vi "Lockin-4461 -Patrick -State 2.0.vi"(10 "IV Curve Mode":bool, 11 "Channels: AO":T8={"AO amp (V)"=[0.0, 0.0, 0.0, 0.0, 0.0, 0.0, 0.0, 0.0], "AO DC (V)"=[0.0, 0.0, 0.0, 0.0, 0.0, 0.0, 0.0, 0.0], "AO f (Hz)"=[13.0, 13.0, 13.0, 13.0, 13.0, 13.0, 13.0, 13.0], "AO phi (deg)"=[0.0, 0.0, 0.0, 0.0, 0.0, 0.0, 0.0, 0.0], "function"=[enum."Sine Wave", enum."Sine Wave", enum."Sine Wave", enum."Sine Wave", enum."Sine Wave", enum."Sine Wave", enum."Sine Wave", enum."Sine Wave"]} {"AO f (Hz)" min=0.001 max=10000.0; "AO DC (V)" format="%#_6p"; "AO amp (V)" format="%#_6p"}) -> ()   [LabVIEW 2013]
uses:
  <vilib>/Analysis/4window.llb/windowTd.ctl
  <vilib>/measure/maspectr.llb/Power Spectrum and PSD Export Mode.ctl
  <vilib>/Utility/error.llb/DialogType.ctl
  <vilib>/Analysis/baseanly.llb/Mean (DBL).vi
  <vilib>/Analysis/2dsp.llb/Decimate (single shot).vi
  <vilib>/Analysis/2dsp.llb/Decimate (single shot, DBL).vi
  <userlib>/_OpenG.lib/array/array.llb/Empty 1D Array (Variant)__ogtk.vi
  <vilib>/Platform/browser.llb/Open URL in Default Browser (string).vi
  <userlib>/_OpenG.lib/error/error.llb/Filter Error Codes (Array)__ogtk.vi
  <userlib>/_OpenG.lib/array/array.llb/Empty 1D Array (DBL)__ogtk.vi
  <vilib>/measure/maspectr.llb/FFT Power Spectrum and PSD for N Chan.vi
  <vilib>/Waveform/WDTOps.llb/WDT Waveform to XY Pairs DBL.vi
  <vilib>/measure/NI_MAPro.lvlib
  <vilib>/Analysis/NI_AALBase.lvlib
  <vilib>/Utility/config.llb/NI_LVConfig.lvlib
  <vilib>/Analysis/NI_AALPro.lvlib
panel:
  in  "Tab Control 3":enum32{"Page 1"}(tab)
  in  "Notes":string
  in  "Path":path=path "C:/Data/lockin"
  in  "EXIT":bool
  in  "RESET":bool
  in  "Save Data":bool
  out "X or R":dbl=0.0008668764236983905 caption="X or R: Current (A) or Voltage (V)" format="%#.3p"
  out "Y or Theta":dbl=-50.403184981183465 caption="Y or Theta: Current (A) or Voltage (V)" format="%.3p"
  in  "Display":enum16{"X and Y", "R and Theta"}(ring)=enum."R and Theta"
  in  "Channel":dbl min=0.0 max=7.0 step=1.0
  in  "Remote Mode":bool
  out "time and date":string="22:19:38.7   2016-11-29"
  out "DAQ mode string":string="None"
  out "time since trigger":dbl
  in  "mean":dbl[](array[numeric])=[0.003634816212724108, -0.004266485588942877, 0.0008988807363483967, 0.001923221656187443, -0.0014081863319705614, 0.0031806607498407746, -0.004900231349882742, 0.00649024630273491]
  in  "Tab Control 2":T1(tab)
  in  "Output signals?":bool
  out "Signals Graph":waveform(dbl)[](graph)=[{"t0"=timestamp(3563320778.6520257 s since 1904-01-01), "dt"=1.0, "Y"=array[10000 elements]}, {"t0"=timestamp(3563320778.6520257 s since 1904-01-01), "dt"=1.0, "Y"=array[10000 elements]}, {"t0"=timestamp(3563320778.6520257 s since 1904-01-01), "dt"=1.0, "Y"=array[10000 elements]}, {"t0"=timestamp(3563320778.6520257 s since 1904-01-01), "dt"=1.0, "Y"=array[10000 elements]}, {"t0"=timestamp(3563320778.6520257 s since 1904-01-01), "dt"=1.0, "Y"=array[10000 elements]}, {"t0"=timestamp(3563320778.6520257 s since 1904-01-01), "dt"=1.0, "Y"=array[10000 elements]}]
  out "Reference Graph":waveform(dbl)[](graph)=[{"t0"=timestamp(3563320778.6520257 s since 1904-01-01), "dt"=1.0, "Y"=array[10000 elements]}, {"t0"=timestamp(3563320778.6520257 s since 1904-01-01), "dt"=1.0, "Y"=array[10000 elements]}]
  in  "decimate graph":i32=1
  in  "Display n?":bool=TRUE
  out "Display X (or R)":waveform(dbl)[](graph)=[{"t0"=timestamp(3563320778.6520257 s since 1904-01-01), "dt"=1.0, "Y"=[0.0008668764236983905]}, {"t0"=timestamp(3563320778.6520257 s since 1904-01-01), "dt"=1.0, "Y"=[0.00020063218028043531]}, {"t0"=timestamp(3563320778.6520257 s since 1904-01-01), "dt"=1.0, "Y"=[0.0004798692615792062]}, {"t0"=timestamp(3563320778.6520257 s since 1904-01-01), "dt"=1.0, "Y"=[0.0003139913967086241]}, {"t0"=timestamp(3563320778.6520257 s since 1904-01-01), "dt"=1.0, "Y"=[0.0013688193701035607]}, {"t0"=timestamp(3563320778.6520257 s since 1904-01-01), "dt"=1.0, "Y"=[0.0007742329964964507]}]
  out "Display Y (or Theta)":waveform(dbl)[](graph)=[{"t0"=timestamp(3563320778.6520257 s since 1904-01-01), "dt"=1.0, "Y"=[-50.403184981183465]}, {"t0"=timestamp(3563320778.6520257 s since 1904-01-01), "dt"=1.0, "Y"=[39.73938237868613]}, {"t0"=timestamp(3563320778.6520257 s since 1904-01-01), "dt"=1.0, "Y"=[21.201240513774476]}, {"t0"=timestamp(3563320778.6520257 s since 1904-01-01), "dt"=1.0, "Y"=[-175.14041289086117]}, {"t0"=timestamp(3563320778.6520257 s since 1904-01-01), "dt"=1.0, "Y"=[12.701682384866178]}, {"t0"=timestamp(3563320778.6520257 s since 1904-01-01), "dt"=1.0, "Y"=[-144.55373858263823]}]
  out "XY Graph":cluster{dbl[], dbl[]}[](graph)=[{[0.0, 0.0005525306980508707], [0.0, -0.0006679704796437707]}, {[0.0, 0.00015427818452350427], [0.0, 0.00012826345365774563]}, {[0.0, 0.00044738977677601506], [0.0, 0.00017354220191319477]}, {[0.0, -0.0003128626906248802], [0.0, -2.6599511687116452e-05]}, {[0.0, 0.0013353217431358285], [0.0, 0.0003009689523512374]}, {[0.0, -0.0006307365060724987], [0.0, -0.0004490080096961856]}]
  out "Results\n(X, Y, R, Theta, mean)":dbl[][](array[numeric])=[[0.0005525306980508707, -0.0006679704796437707, 0.0008668764236983905, -50.403184981183465, 0.0012252162534641732], [0.00015427818452350427, 0.00012826345365774563, 0.00020063218028043531, 39.73938237868613, -0.005160459243691849], [0.00044738977677601506, 0.00017354220191319477, 0.0004798692615792062, 21.201240513774476, -0.0026575626784062123], [-0.0003128626906248802, -2.6599511687116452e-05, 0.0003139913967086241, -175.14041289086117, 0.0015251935804346806], [0.0013353217431358285, 0.0003009689523512374, 0.0013688193701035607, 12.701682384866178, -0.0022716878303714787], [-0.0006307365060724987, -0.0004490080096961856, 0.0007742329964964507, -144.55373858263823, -0.006832938051437891], [0.0, 0.0, 0.0, 0.0, -0.00026027857304379033], [0.0, 0.0, 0.0, 0.0, 0.0008661123672393431]] format="%#_3p"
  out "PS Chart":dbl[][](graph)=[[-1411.497616925462, -1404.3790029743438, -1413.0961920610762, -1418.6418791322994, -1413.136726104145, -1413.4151534226191, -1417.9246313001065, -1424.6072395567076]]
  out "PS dB":cluster{"f0":dbl, "df":dbl, "magnitude":dbl[]}[](graph)
  in  "window":T2=1 items=["Rectangle"=0, "Hanning"=1, "Hamming"=2, "Blackman-Harris"=3, "Exact Blackman"=4, "Blackman"=5, "Flat Top"=6, "4 Term B-Harris "=7, "7 Term B-Harris"=8, "Low Sidelobe"=9, "Blackman Nuttall"=11, "Triangle"=30, "Bartlett-Hanning"=31, "Bohman"=32, "Parzen"=33, "Welch"=34, "Kaiser"=60, "Dolph-Chebyshev"=61, "Gaussian"=62]
  in  "averaging parameters":T3={"averaging mode"=enum."RMS averaging", "weighting mode"=enum."Exponential", "number of averages"=10} {"number of averages" min=1}
  in  "restart averaging (F)":bool
  in  "export mode":T4 items=["Power Spectrum", "Power Spectral Density"]
  in  "window parameter":dbl=nan
  out "averages\ncompleted":dbl=8319.0
  out "averaging done":bool=TRUE
  in  "Tab Control":T5(tab)=enum."AO/Lockin Setup"
  in  "save config":bool
  in  "load config":bool
  in  "Instrument":u16(ring) items=["SIMULATE", "CF900", "DR200", "MNK", "PPMS1", "PPMS2", "THz1", "THz2"]
  in  "AO Configuration":T6(array[cluster])
  in  "AI Configuration":T7(array[cluster])
  in  "#s":i32=10000
  in  "Fs":i32=130000
  in  "auto size":bool=TRUE
  in  "decimating factor":i32=1
  in  "AI Buffer Size (S)":i32=100
  out "dt":dbl=7.692307692307692e-06 format="%#_6p"
  in  "frequency multiplier":dbl=10000.0 format="%#_13g"
  out "sampling info":cluster{"Fs":i32, "#s":i32}={"Fs"=4000, "#s"=10000}
  in  "DAQ Type":enum16{"None", "USB 4431", "PXI 446x"}(ring)
  in  "Amplifiers":enum16{"None", "Krohn Hite", "Femto"}(ring)
  in  "...............reset REF":bool
  in  "............zero offset":bool
  in  "....measure offset":bool
  in  "............all  f same":bool
  in  "..........reset signal":bool
  in  "60 Hz prefilter":bool
  in  "LP prefilter":bool
  in  "LP cutoff (Hz)":dbl=30.0
  in  "Channels: Lockin":T9={"REF f (Hz)"=[13.0], "REF phi (deg)"=[0.0]} {"REF phi (deg)" format="%#_3g"}
  in  "D":dbl=0.019999999999999997 format="%.2f"
  in  "I":dbl=0.6 format="%.2f"
  in  "P":dbl=0.5 format="%.2f"
  in  "autophase?\n(experimental)":bool
  out "filter fC (Hz)":dbl=0.5305164769729844
  in  "TC (s)":dbl=0.3 format="%#_6p"
  in  "order":i32=2
  out "Current State":string
  out "State History":string
  in  "offsets":dbl[](array[numeric])=[-2.856912612915039e-05, 0.0001668522834777832, 0.00010829269886016845, 0.0027965894103050234, 0.002931471037864685, 0.0029329052329063418] format="%#.2p"
  in  "Gain":dbl[](array[numeric])=[1.0, 1.0, 1.0, 1.0, 1.0, 1.0, 1.0, 1.0]
  out "phase log":dbl[](array[numeric])=[357.0, 357.0, 357.0, 357.0, 357.0, 357.0, 357.0, 357.0] format="%.1f"
  out "AI tasks":i32
  out "AO tasks":i32
  in  "Bug":bool
  out "error":errorcluster
  # "´"
  # "Multichannel Lockin v2016/12/12 v2.0"
  # "plot 0    = AI0 f0\nplot 1    = Ai1 f0\n...\nplot N-1  = AIN f0\n\nplot N    = AI0 f1\nplot N+1  = AI1 f1\n..."
  # "configuration"
  # "sampling"
  # "AO Settings"
  # "Lockin Settings"
  # "prefilters"
  # "lockin filter"
  # "autophase"
  # "0"
  # "1"
  # "2"
  # "3"
  # "4"
  # "5"
  # "6"
  # "7"
  # "Or send an email p.irvin@levylab.org\nwith questions or suggestions."
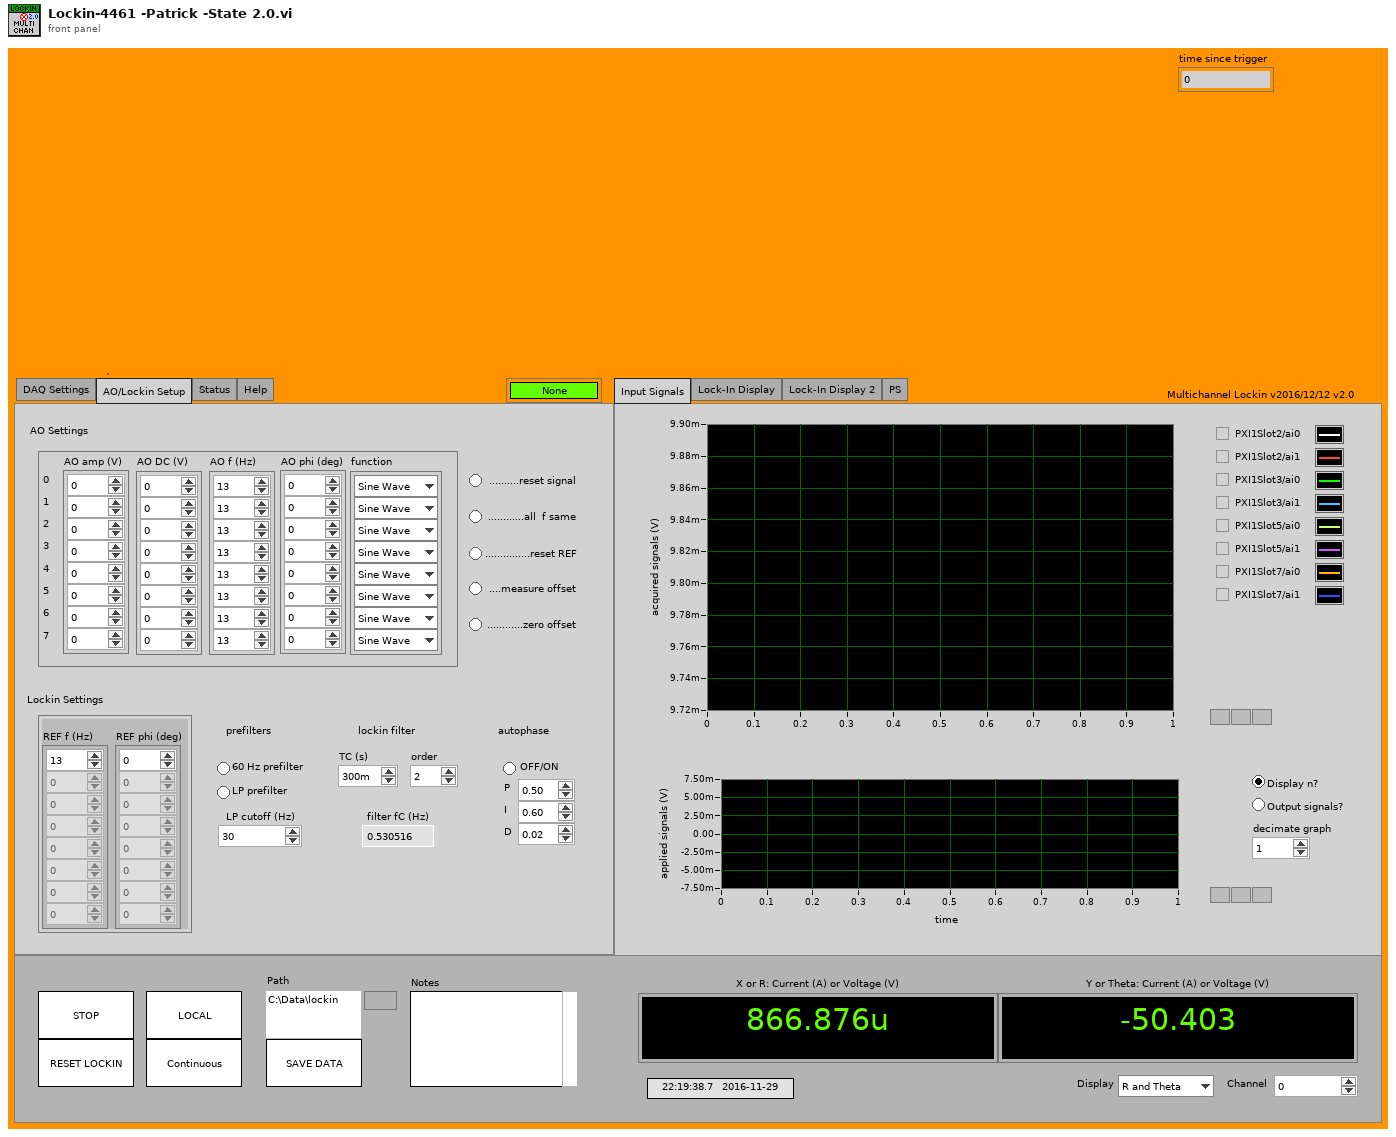
[diagram p1: front panel]
types:
  T1 = enum32{"Input Signals", "Lock-In Display", "Lock-In Display 2", "PS"}
  T2 = typedef "NI_AALPro.lvlib/windowTd.ctl" = u32
  T3 = cluster{"averaging mode":enum16{"No averaging", "Vector averaging", "RMS averaging", "Peak hold"}, "weighting mode":enum16{"Linear", "Exponential"}, "number of averages":u32}
  T4 = typedef "NI_MAPro.lvlib/Power Spectrum and PSD Export Mode.ctl" = u16
  T5 = enum32{"DAQ Settings", "AO/Lockin Setup", "Status", "Help"}
  T6 = cluster{"Output physical channels":tag, "AO. Max":dbl, "AO.Min":dbl}[]
  T7 = cluster{"AI.Coupling":enum16{"AC", "DC", "GND"}, "AI.Max":dbl, "AI.Min":dbl, "Input physical channels":tag}[]
  T8 = cluster{"AO amp (V)":dbl[], "AO DC (V)":dbl[], "AO f (Hz)":dbl[], "AO phi (deg)":dbl[], "function":enum16{"Sine Wave", "Triangle Wave", "Square Wave", "Sawtooth Wave"}[]}
  T9 = cluster{"REF f (Hz)":dbl[], "REF phi (deg)":dbl[]}
  T10 = enum32{"invalid app kind", "Development System", "Run Time System", "Student Edition", "Embedded LabVIEW", "Evaluation", "Custom"}
  T11 = enum32{"Invalid", "Standard", "Closed", "Hidden", "Minimized", "Maximized"}
  T12 = enum32{"Input Signals", "Lock-In Display", "Lock-In Display 2", "PS", "FFT"}
  T13 = cluster{"Core":cluster{"Current VI Reference":refnum<vi>, "Close Panel on Exit?":bool}, "Error":bool, "Your string data":string, "AI task":refnum<k21>[], "AO task":refnum<k21>[], "Input Signals":waveform(dbl)[], "Ouput Signals":waveform(dbl)[], "REF":waveform(dbl)[], "sampling info":cluster{"Fs":dbl, "#s":dbl}, "Tasks":string[]}
  T14 = typedef "DialogType.ctl" = u16
  T15 = cluster{"Current VI Reference":refnum<vi>, "Close Panel on Exit?":bool}
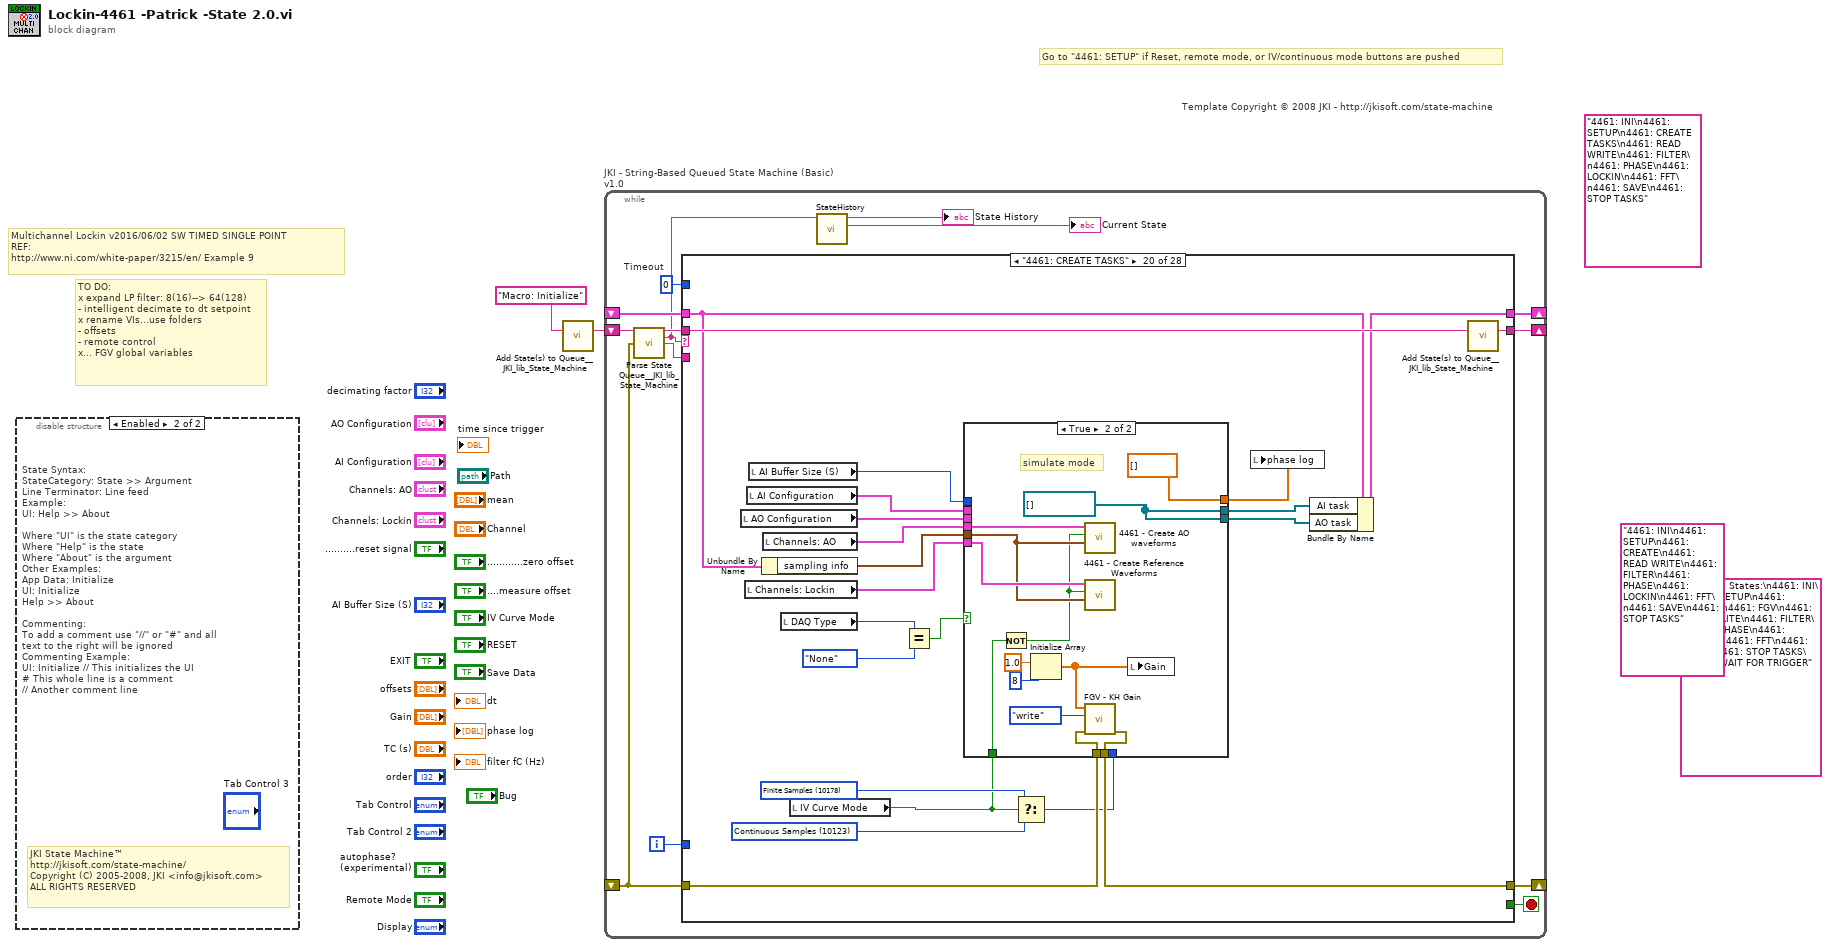
[diagram p0: block diagram]
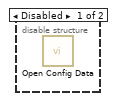
[diagram p2: hidden frame]
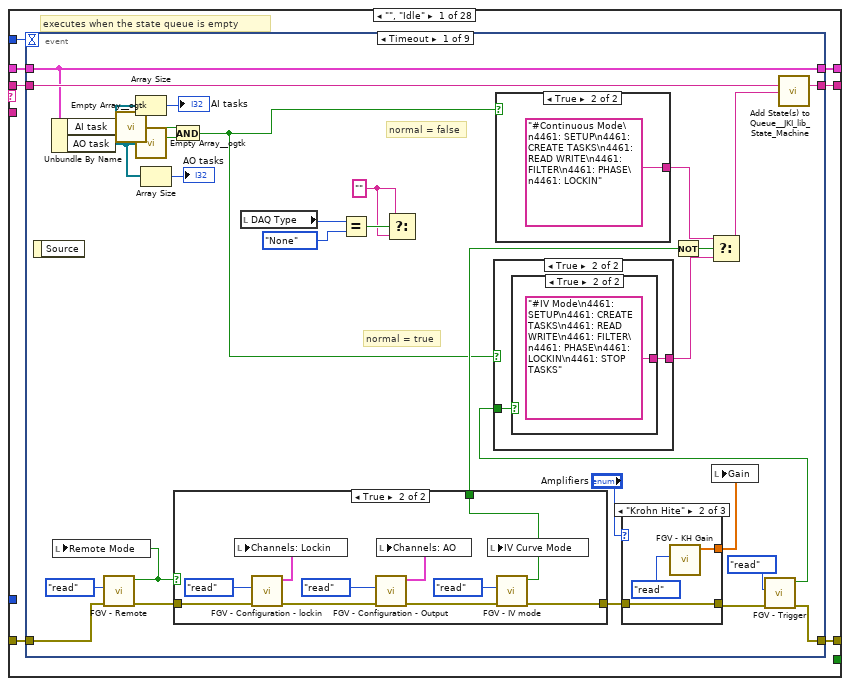
[diagram p3: hidden frame]
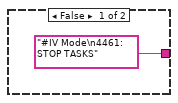
[diagram p4: hidden frame]
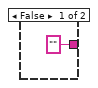
[diagram p5: hidden frame]
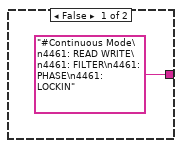
[diagram p6: hidden frame]
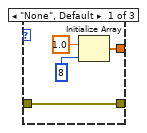
[diagram p7: hidden frame]
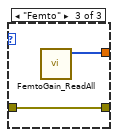
[diagram p8: hidden frame]
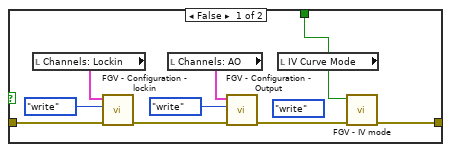
[diagram p9: hidden frame]
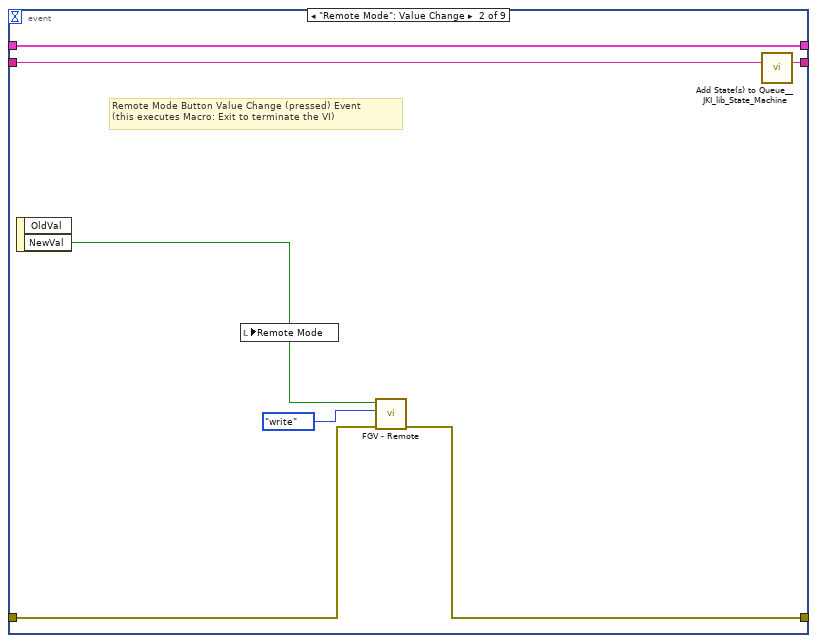
[diagram p10: hidden frame]
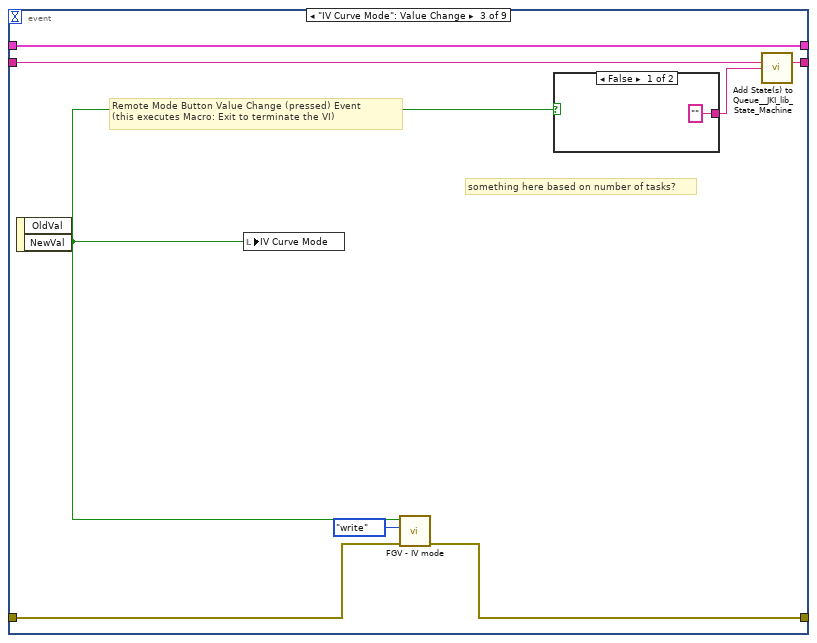
[diagram p11: hidden frame]
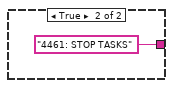
[diagram p12: hidden frame]
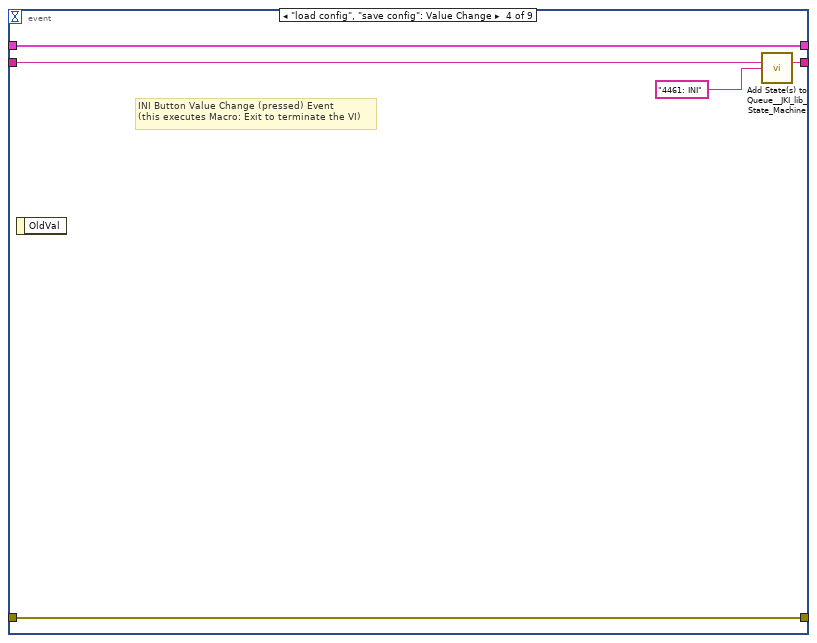
[diagram p13: hidden frame]
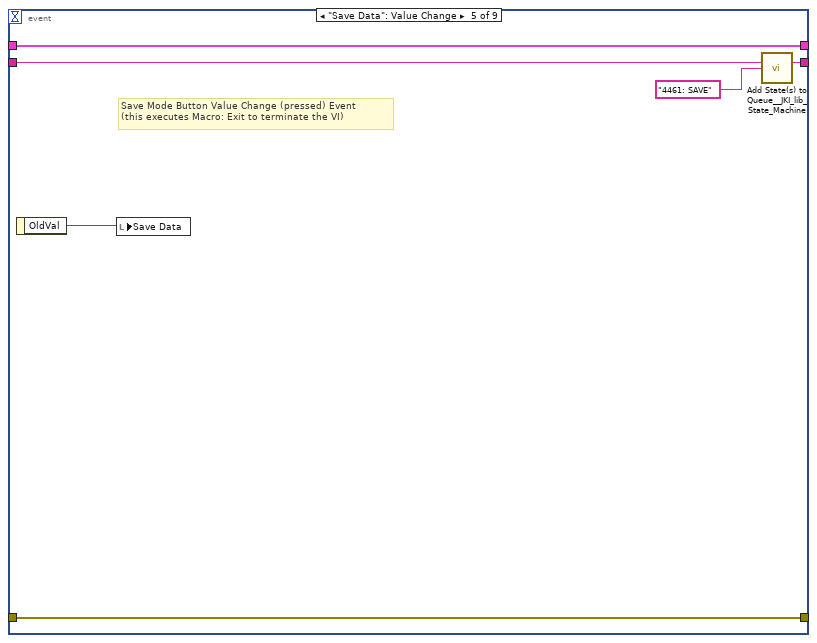
[diagram p14: hidden frame]
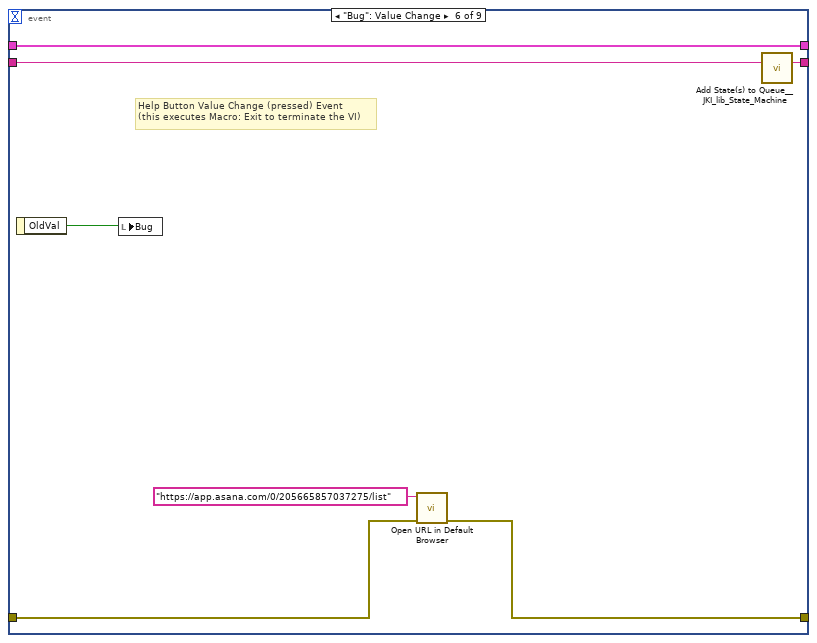
[diagram p15: hidden frame]
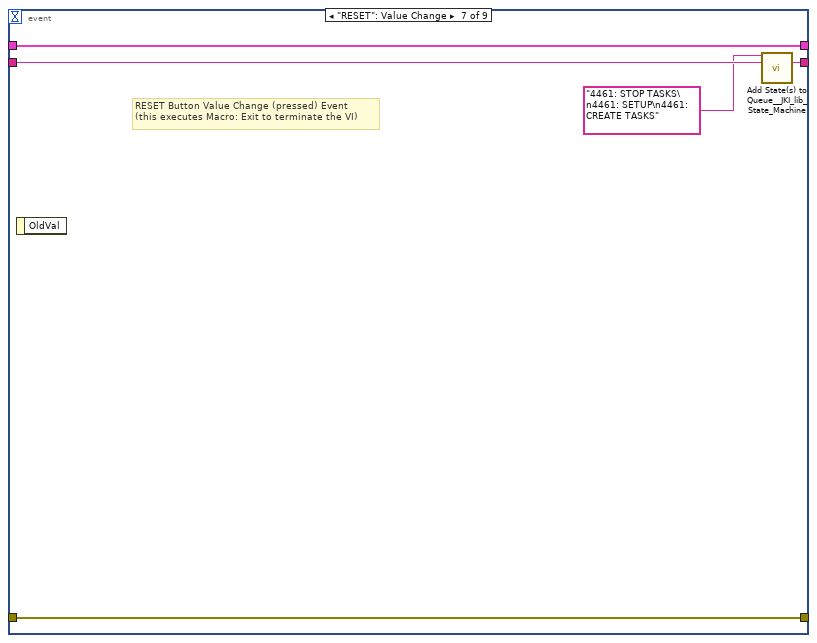
[diagram p16: hidden frame]
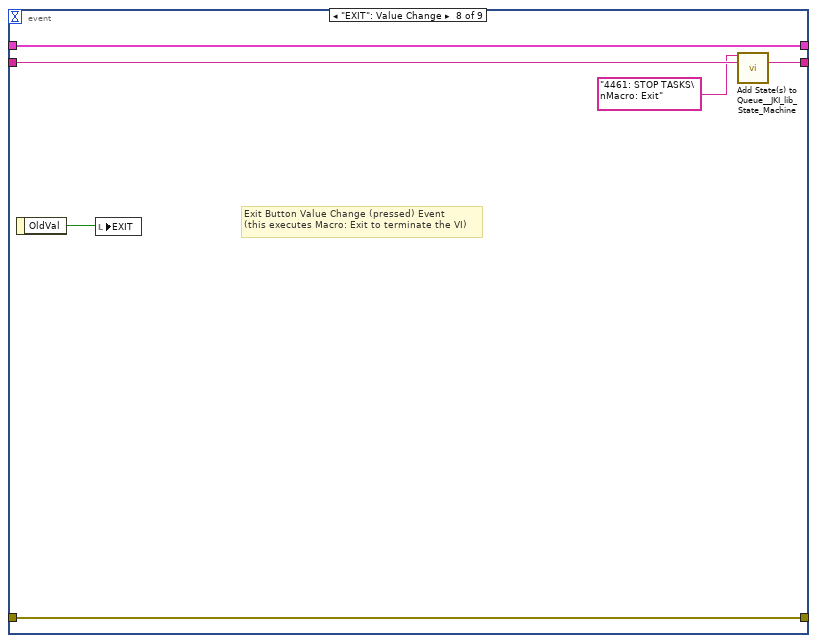
[diagram p17: hidden frame]
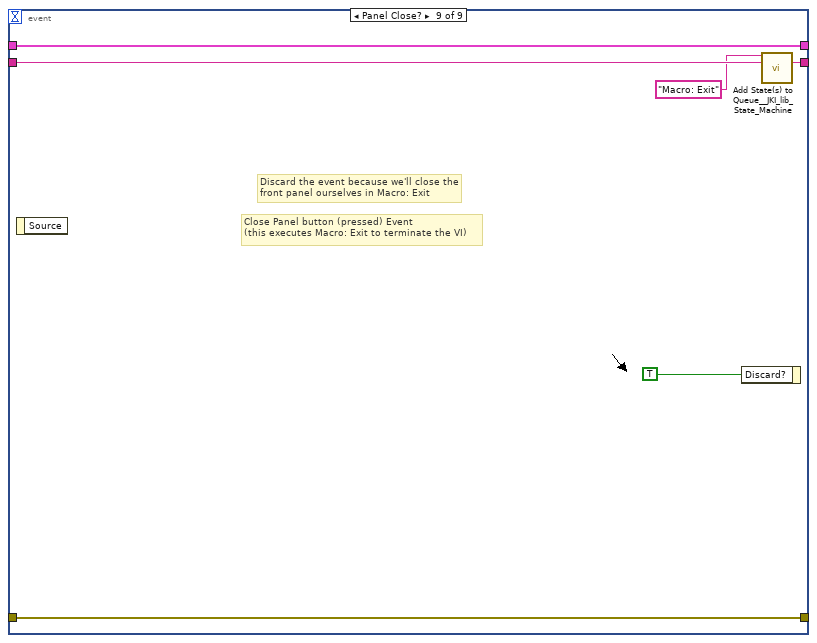
[diagram p18: hidden frame]
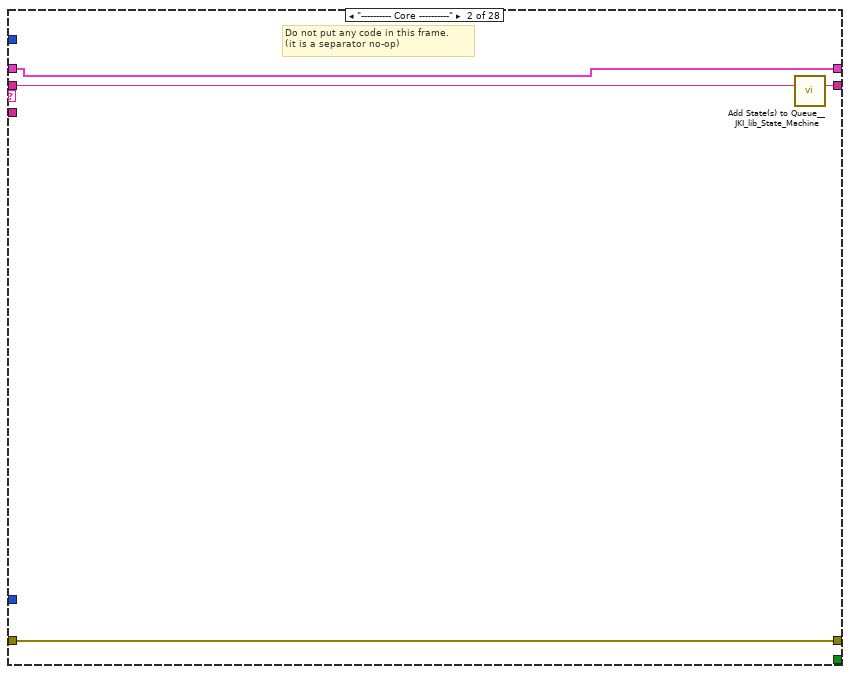
[diagram p19: hidden frame]
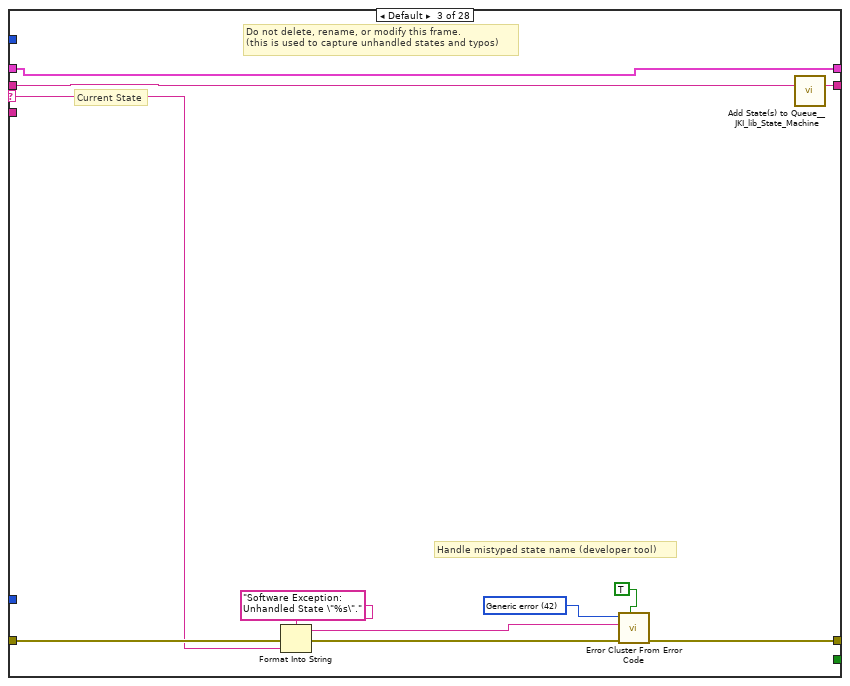
[diagram p20: hidden frame]
diagram:
  (unwired) "4461: INI\n4461: SETUP\n4461: CREATE\n4461: READ WRITE\n4461: FILTER\n4461: PHASE\n4461: LOCKIN\n4461: FFT\n4461: SAVE\n4461: STOP TASKS" ("State(s) at Back (\"\")")
  (unwired) "All 4461 States:\n4461: INI\n4461: SETUP\n4461: CREATE\n4461: FGV\n4461: READ WRITE\n4461: FILTER\n4461: PHASE\n4461: LOCKIN\n4461: FFT\n4461: SAVE\n4461: STOP TASKS\n4461: WAIT FOR TRIGGER" ("State(s) at Back (\"\")")
  (unwired) "4461: INI\n4461: SETUP\n4461: CREATE TASKS\n4461: READ WRITE\n4461: FILTER\n4461: PHASE\n4461: LOCKIN\n4461: FFT\n4461: SAVE\n4461: STOP TASKS" ("State(s) at Back (\"\")")
  # "Template Copyright © 2008 JKI - http://jkisoft.com/state-machine"
  # "Go to \"4461: SETUP\" if Reset, remote mode, or IV/continuous mode buttons are pushed"
  # "Multichannel Lockin v2016/06/02 SW TIMED SINGLE POINT\nREF:\nhttp://www.ni.com/white-paper/3215/en/ Example 9"
  # "TO DO:\nx expand LP filter: 8(16)--> 64(128)\n- intelligent decimate to dt setpoint\nx rename VIs...use folders\n- offsets\n- remote control\nx... FGV global variables"
  n1 = disable-structure shown="Enabled" {
    frame Disabled {
      n2 = call <vilib>:"Open Config Data.vi"() -> ()  [unwired: 9 in, 3 out]
    }
    frame Enabled {
      # "JKI State Machine™\nhttp://jkisoft.com/state-machine/\nCopyright (C) 2005-2008, JKI <info@jkisoft.com>\nALL RIGHTS RESERVED"
      # "State Syntax:\nStateCategory: State >> Argument\nLine Terminator: Line feed\nExample:\nUI: Help >> About\n\nWhere \"UI\" is the state category\nWhere \"Help\" is the state\nWhere \"About\" is the argument\nOther Examples:\nApp Data: Initialize\nUI: Initialize\nHelp >> About\n\nCommenting:\nTo add a comment use \"//\" or \"#\" and all text to the right will be ignored\nCommenting Example:\nUI: Initialize // This initializes the UI\n# This whole line is a comment\n// Another comment line"
    }
  }
  n3 = call <vilib>:"Add State(s) to Queue__JKI_lib_State_Machine.vi"("State(s) in (\"\")"="Macro: Initialize") -> ("States Out"=w2:string)  [unwired: 14 in]
  n4 = while "JKI - String-Based Queued State Machine (Basic) v1.0" {
    shift-right: [w5] -> _
    shift-left: _ -> [w6]
    shift-right: [w15] -> _
    shift-left: _ -> [w7]
    shift-right: [w14] -> _
    shift-left: w2 -> [w8]
    i -> [w10]
    stop <- w13 stop-if-true
    w12 = 0  # Timeout
    n5 = call <vilib>:"Parse State Queue__JKI_lib_State_Machine.vi"("State Queue"=w8, "Error In (no error)"=w7) -> ("Remaining States"=w11:string, "Current State"=w3:string, "Arguments"=w16:string)  [unwired: 11 in]
    n6 = case shown="\"4461: CREATE TASKS\"" w3 {
      selector: w3 -> [_ _ w145 _ _ _ _ _ _ _ _ _ _ _ _ _ _ _ _ _ _ _ _ _ _ _ _ _]
      tunnel: w16 -> [_ _ _ _ _ _ _ _ _ _ _ w224 w235 _ _ _ _ _ _ _ _ _ _ _ _ _ _ _]
      tunnel: w6 -> [w21 w141 w147 w158 w173 w185 w188 _ w206 w212 w219 w223 w234 w262 w266 w271 w282 w291 w332 w371 w452 w501 w556 w619 w642 w690 w717 w767]
      tunnel: [w20 w142 w151 w164 errorcluster {"status"=FALSE, "code"=0, "source"=""} ("error out") w184 w189 w202 w207 w213 w217 w225 w233 w263 w268 w279 w283 w288 w321 w373 w460 w512 w545 w620 w644 w680 w718 w766] -> w15
      tunnel: w7 -> [w19 w142 w150 w164 w170 w184 w189 w202 w208 w213 w217 w226 w237 w263 w268 w279 w283 w289 w321 w377 w462 w515 w545 w620 w644 w679 w729 w766]
      tunnel: [w22 w143 w148 w166 w177 w186 w190 w204 w210 w214 w221 w227 w238 w264 w269 w280 w284 w293 w335 w383 w464 w523 w557 w618 w643 w691 w714 w764] -> w14
      tunnel: [_ _ _ _ _ TRUE _ _ _ _ _ _ _ _ _ _ _ _ _ _ _ _ _ _ _ _ _ _] -> w13
      tunnel: [w18 w141 w147 w165 w174 w185 w188 w203 w206 w212 w219 w223 w234 w262 w266 w271 w282 w291 w330 w378 w463 w522 w556 w619 w642 w690 w716 w767] -> w5
      tunnel: w12 -> [w17 _ _ _ _ _ _ _ _ _ _ _ _ _ _ _ _ _ _ _ _ _ _ _ _ _ _ _]
      tunnel: w11 -> [w23 w144 w149 w167 w178 w187 w191 w205 w211 w215 w222 w228 w239 w265 w270 w281 w285 w292 w336 w384 w465 w524 w558 w621 w645 w692 w730 w768]
      tunnel: w10 -> [_ _ _ _ _ _ _ _ _ _ _ _ _ _ _ _ _ _ _ _ _ _ _ _ _ _ _ _]
      frame "", "Idle" {
        # "executes when the state queue is empty"
        n7 = event shown="[0] Timeout" {
          selector: _ -> [_ _ _ _ _ _ _ _ _]
          dyn-events: _ -> [_ _ _ _ _ _ _ _ _]
          timeout: w17 -> [_ _ _ _ _ _ _ _ _]
          tunnel: w23 -> [w53 w95 w103 w110 w116 w123 w128 w134 w140]
          tunnel: [w52 w94 w102 w109 w115 w122 w127 w133 w139] -> w22
          tunnel: w21 -> [w40 w93 w101 w108 w114 w121 w126 w131 w137]
          tunnel: [w41 w90 w98 w106 w113 w118 w125 w132 w138] -> w20
          tunnel: w19 -> [w50 w91 w99 w106 w113 w120 w125 w132 w138]
          tunnel: [w40 w93 w101 w108 w114 w121 w126 w131 w137] -> w18
          event Timeout {
            w25 = "" ("State(s) at Back (\"\")")
            # "normal = true"
            # "normal = false"
            n8 = event-data() -> ()  [unwired: 1 in, 1 out]
            n9 = Unbundle By Name(w40) -> ("AI task"=w32:refnum<k21>[], "AO task"=w30:refnum<k21>[])
            n10 = call "FGV - Remote.vi"("error in"=w50, "Function"=enum16{"write", "read"}."read") -> ("error out"=w48:errorcluster, "Remote Mode"=w43:bool)  [unwired: 4 in]
            n11 = local write "Remote Mode"(w43) -> ()
            n12 = call-poly <userlib>:"Empty Array__ogtk.vi"("Array"=w32) -> ("Empty Array?"=w39:bool)  [unwired: 8 in]
            n13 = Array Size(array=w32) -> (size(s)=→"AI tasks":i32)
            n14 = call-poly <userlib>:"Empty Array__ogtk.vi"("Array"=w30) -> ("Empty Array?"=w38:bool)  [unwired: 8 in]
            n15 = Array Size(array=w30) -> (size(s)=→"AO tasks":i32)
            n16 = And(x=w39, y=w38) -> (x .and. y?=w26:bool)
            n17 = case shown="True" w43 {
              tunnel: [w72 w82] -> w47
              tunnel: w48 -> [w74 w85]
              tunnel: [w70 w79] -> w46
              frame False {
                (unwired) enum16{"write", "read"}."write" ("Function")
                n18 = local read "Channels: Lockin"() -> (w75:T9)
                n19 = call "FGV - Configuration - lockin.vi"("error in"=w74, "Function"=enum16{"write", "read"}."write", "Channels: Lockin"=w75) -> ("error out"=w76:errorcluster)  [unwired: 3 in, 1 out]
                n20 = local read "Channels: AO"() -> (w71:T8)
                n21 = call "FGV - Configuration - Output.vi"("error in"=w76, "Function"=enum16{"write", "read"}."write", "Channels: AO"=w71) -> ("error out"=w73:errorcluster)  [unwired: 3 in, 1 out]
                n22 = local read "IV Curve Mode"() -> (w70:bool)
                n23 = call "FGV - IV mode.vi"("error in"=w73, "IV mode"=w70) -> ("error out"=w72:errorcluster)  [unwired: 4 in, 1 out]
              }
              frame True {
                n24 = call "FGV - Configuration - lockin.vi"("error in"=w85, "Function"=enum16{"write", "read"}."read") -> ("error out"=w86:errorcluster, "Channels: Lockin 2"=w84:T9)  [unwired: 4 in]
                n25 = local write "Channels: Lockin"(w84) -> ()
                n26 = call "FGV - Configuration - Output.vi"("error in"=w86, "Function"=enum16{"write", "read"}."read") -> ("error out"=w83:errorcluster, "Channels: AO 2"=w81:T8)  [unwired: 4 in]
                n27 = local write "Channels: AO"(w81) -> ()
                n28 = call "FGV - IV mode.vi"("error in"=w83, "Function"=enum16{"write", "read"}."read") -> ("error out"=w82:errorcluster, "IV mode"=w79:bool)  [unwired: 4 in]
                n29 = local write "IV Curve Mode"(w79) -> ()
              }
            }
            n30 = local read "DAQ Type"() -> (w35:enum16{"None", "USB 4431", "PXI 446x"})
            n31 = Equal?(x=w35, y=enum16{"None", "USB 4431", "PXI 446x"}."None" ("DAQ Type")) -> (x = y?=w33:bool)
            n32 = Select(t=w25, s=w33, f=w25) -> ()  [unwired: 1 out]
            n33 = case shown="True" w26 {
              tunnel: ["#Continuous Mode\n4461: READ WRITE\n4461: FILTER\n4461: PHASE\n4461: LOCKIN" ("State(s) at Back (\"\")") "#Continuous Mode\n4461: SETUP\n4461: CREATE TASKS\n4461: READ WRITE\n4461: FILTER\n4461: PHASE\n4461: LOCKIN" ("State(s) at Back (\"\")")] -> w28
              frame False {
              }
              frame True {
              }
            }
            n34 = case shown="\"Krohn Hite\"" "Amplifiers" {
              tunnel: [w62 w67 w68] -> w42
              tunnel: [w63 w66 w69] -> w49
              tunnel: w47 -> [w62 w67 w68]
              frame "None", Default {
                n35 = Initialize Array(1.0 ("element"), 8 ("dimension size")) -> (w63:dbl[])
              }
              frame "Krohn Hite" {
                n36 = call <userlib>:"FGV - KH Gain.vi"("Function"=enum16{"write", "read"}."read") -> ("Array 2"=w66:dbl[])  [unwired: 5 in, 1 out]
              }
              frame "Femto" {
                n37 = call <userlib>:"FemtoGain_ReadAll.vi"() -> ("Femto Gains"=w69:i32[])  [unwired: 11 in]
              }
            }
            n38 = Not(x=w46) -> (.not. x?=w36:bool)
            n39 = local write "Gain"(w49) -> ()
            n40 = call "FGV - Trigger.vi"("error in"=w42, "Function"=enum16{"write", "read"}."read") -> ("error out"=w41:errorcluster, "Trigger 2"=w27:bool)  [unwired: 4 in]
            n41 = case shown="True" w26 {
              tunnel: ["#IV Mode\n4461: STOP TASKS" ("State(s) at Back (\"\")") w56] -> w44
              tunnel: w27 -> [_ w55]
              frame False {
              }
              frame True {
                n42 = case shown="True" w55 {
                  tunnel: ["" ("State(s) at Back (\"\")") "#IV Mode\n4461: SETUP\n4461: CREATE TASKS\n4461: READ WRITE\n4461: FILTER\n4461: PHASE\n4461: LOCKIN\n4461: STOP TASKS" ("State(s) at Back (\"\")")] -> w56
                  frame False {
                  }
                  frame True {
                  }
                }
              }
            }
            n43 = Select(t=w28, s=w36, f=w44) -> (s? t:f=w37:string)
            n44 = call <vilib>:"Add State(s) to Queue__JKI_lib_State_Machine.vi"("State(s) in (\"\")"=w53, "State(s) at Back (\"\")"=w37) -> ("States Out"=w52:string)  [unwired: 13 in]
          }
          event "Remote Mode": Value Change {
            # "Remote Mode Button Value Change (pressed) Event\n(this executes Macro: Exit to terminate the VI)"
            n45 = event-data() -> ("NewVal"=w89:bool)  [unwired: 1 in, 1 out]
            n46 = local write "Remote Mode"(w89) -> ()
            n47 = call "FGV - Remote.vi"("error in"=w91, "Function"=enum16{"write", "read"}."write", "Remote Mode"=w89) -> ("error out"=w90:errorcluster)  [unwired: 3 in, 1 out]
            n48 = call <vilib>:"Add State(s) to Queue__JKI_lib_State_Machine.vi"("State(s) in (\"\")"=w95) -> ("States Out"=w94:string)  [unwired: 14 in]
          }
          event "IV Curve Mode": Value Change {
            # "something here based on number of tasks?"
            # "Remote Mode Button Value Change (pressed) Event\n(this executes Macro: Exit to terminate the VI)"
            n49 = event-data() -> ("NewVal"=w96:bool)  [unwired: 1 in, 1 out]
            n50 = local write "IV Curve Mode"(w96) -> ()
            n51 = call "FGV - IV mode.vi"("error in"=w99, "Function"=enum16{"write", "read"}."write", "IV mode"=w96) -> ("error out"=w98:errorcluster)  [unwired: 3 in, 1 out]
            n52 = case shown="False" w96 {
              tunnel: ["" ("State(s) at Back (\"\")") "4461: STOP TASKS" ("State(s) at Back (\"\")")] -> w97
              frame False {
              }
              frame True {
              }
            }
            n53 = call <vilib>:"Add State(s) to Queue__JKI_lib_State_Machine.vi"("State(s) in (\"\")"=w103, "State(s) at Back (\"\")"=w97) -> ("States Out"=w102:string)  [unwired: 13 in]
          }
          event "load config", "save config": Value Change {
            # "INI Button Value Change (pressed) Event\n(this executes Macro: Exit to terminate the VI)"
            n54 = event-data() -> ()  [unwired: 1 in, 1 out]
            n55 = call <vilib>:"Add State(s) to Queue__JKI_lib_State_Machine.vi"("State(s) in (\"\")"=w110, "State(s) at Back (\"\")"="4461: INI") -> ("States Out"=w109:string)  [unwired: 13 in]
          }
          event "Save Data": Value Change {
            # "Save Mode Button Value Change (pressed) Event\n(this executes Macro: Exit to terminate the VI)"
            n56 = event-data() -> ("OldVal"=w111:bool)  [unwired: 1 in]
            n57 = local write "Save Data"(w111) -> ()
            n58 = call <vilib>:"Add State(s) to Queue__JKI_lib_State_Machine.vi"("State(s) in (\"\")"=w116, "State(s) at Back (\"\")"="4461: SAVE") -> ("States Out"=w115:string)  [unwired: 13 in]
          }
          event "Bug": Value Change {
            # "Help Button Value Change (pressed) Event\n(this executes Macro: Exit to terminate the VI)"
            n59 = event-data() -> ("OldVal"=w117:bool)  [unwired: 1 in]
            n60 = local write "Bug"(w117) -> ()
            n61 = call-poly <vilib>:"Open URL in Default Browser.vi"("error in (no error)"=w120, "URL"="https://app.asana.com/0/205665857037275/list") -> ("error out"=w118:errorcluster)  [unwired: 4 in, 1 out]
            n62 = call <vilib>:"Add State(s) to Queue__JKI_lib_State_Machine.vi"("State(s) in (\"\")"=w123) -> ("States Out"=w122:string)  [unwired: 14 in]
          }
          event "RESET": Value Change {
            # "RESET Button Value Change (pressed) Event\n(this executes Macro: Exit to terminate the VI)"
            n63 = event-data() -> ()  [unwired: 1 in, 1 out]
            n64 = call <vilib>:"Add State(s) to Queue__JKI_lib_State_Machine.vi"("State(s) in Front (\"\")"="4461: STOP TASKS\n4461: SETUP\n4461: CREATE TASKS", "State(s) in (\"\")"=w128) -> ("States Out"=w127:string)  [unwired: 13 in]
          }
          event "EXIT": Value Change {
            # "Exit Button Value Change (pressed) Event\n(this executes Macro: Exit to terminate the VI)"
            n65 = event-data() -> ("OldVal"=w129:bool)  [unwired: 1 in]
            n66 = local write "EXIT"(w129) -> ()
            n67 = call <vilib>:"Add State(s) to Queue__JKI_lib_State_Machine.vi"("State(s) in Front (\"\")"="4461: STOP TASKS\nMacro: Exit", "State(s) in (\"\")"=w134) -> ("States Out"=w133:string)  [unwired: 13 in]
          }
          event Panel Close? {
            # "Discard the event because we'll close the front panel ourselves in Macro: Exit"
            # "Close Panel button (pressed) Event\n(this executes Macro: Exit to terminate the VI)"
            n68 = event-data() -> ()  [unwired: 1 in, 1 out]
            n69 = event-data("Discard?"=TRUE) -> ()  [unwired: 1 in, 1 out]
            n70 = call <vilib>:"Add State(s) to Queue__JKI_lib_State_Machine.vi"("State(s) in Front (\"\")"="Macro: Exit", "State(s) in (\"\")"=w140) -> ("States Out"=w139:string)  [unwired: 13 in]
          }
        }
      }
      frame "---------- Core ----------" {
        # "Do not put any code in this frame.\n(it is a separator no-op)"
        n71 = call <vilib>:"Add State(s) to Queue__JKI_lib_State_Machine.vi"("State(s) in (\"\")"=w144) -> ("States Out"=w143:string)  [unwired: 14 in]
      }
      frame Default {
        w154 = 42 items=["No error", "Argument error", "Memory is full", "Out of zone", "End of file", "File already open", "Generic file I/O error", "File not found", "File permission error", "Disk is full", "Duplicate path", "Too many files open", "System feature not enabled", "Resource file not found", "Cannot add resource", "Resource not found", "Image not found", "Image memory error", "Pen does not exist", "Config type invalid", "Config token not found", "Config parse error", "Config memory error", "Bad external code format", "Bad external code offset", "External code not present", "Null window", "Destroy window error", "Null menu", "Print aborted", "Bad print record", "Print driver error", "Windows error during printing", "Memory error during printing", "Print dialog error", "Generic print error", "Invalid device refnum", "Device not found", "Device parameter error", "Device unit error", "Cannot open device", "Device call aborted", "Generic error", "Cancelled by user", "Object ID too low", "Object ID too high", "Object not in heap", "Unknown heap", "Unknown object (invalid DefProc)", "Unknown object (DefProc not in table)", "Message out of range", "Invalid (null) method", "Unknown message", "Manager call not supported", "Bad address", "Network operation in progress", "Network operation timed out", "Connection is busy", "Network attribute not supported", "Network error", "Address in use", "System out of memory", "Connection aborted", "Connection refused", "Not connected", "Already connected", "Connection closed", "Initialization error (interapplication manager)", "Bad occurrence", "Wait on unbound occurrence handler", "Occurrence queue overflow", "Datalog type conflict", "Unused", "Unrecognized type (interapplication manager)", "Memory corrupt", "Failed to make temporary DLL", "Old CIN version", "Drag socket not found", "Failed to load drop-object", "Failed to register OLE object", "Failed to release OLE object", "Format specifier type mismatch", "Unknown format specifier", "Too few format specifiers", "Too many format specifiers", "Scan failed", "Newer CIN version", "Error converting to variant", "Runtime menu error", "Password tampered", "Variant attribute not found", "Incompatible variant data type", "Event data is not available", "Event Store is not present", "Occurrence is not found", "Event Queue is not created", "Event info is not available", "Refnum passed is NULL", "Error retrieving Class GUID", "Error retrieving CoClass GUID", "Error retrieving TypeLib GUID.", "Bad built application magic bytes.", "Specific driver is different from the specific driver associated with the Logical Name.", "There is no session opened to the class driver.", "Max Error", "MAX - Error with config objects", "MAX - Error loading configuration", "MAX - Group not supported"]
        # "Current State"
        # "Do not delete, rename, or modify this frame.\n(this is used to capture unhandled states and typos)"
        # "Handle mistyped state name (developer tool)"
        n72 = Format Into String(format string="Software Exception: Unhandled State \"%s\"." ("message"), error in=w150, w145) -> (resulting string=w153:string, error out=w152:errorcluster)  [unwired: 1 in]
        n73 = call <vilib>:"Error Cluster From Error Code.vi"("show call chain? (False)"=TRUE, "error in (no error)"=w152, "error message (\"\")"=w153, "error code (0)"=w154) -> ("error out"=w151:errorcluster)  [unwired: 5 in]
        n74 = call <vilib>:"Add State(s) to Queue__JKI_lib_State_Machine.vi"("State(s) in (\"\")"=w149) -> ("States Out"=w148:string)  [unwired: 14 in]
      }
      frame "Initialize Core Data" {
        # "Do not delete, rename, or modify this frame.\n(this is used to determine panel behavior on exit)"
        # "originally closed?"
        # "exe?"
        # "If panel starts closed or is an EXE, then close it when we exit"
        n75 = property class="VI"() -> ("Front Panel.Open"=w163:bool)  [unwired: 2 in, 2 out]
        n76 = property class="App"() -> ("App.Kind"=w162:T10)  [unwired: 2 in, 2 out]
        n77 = control-ref of="Current VI Reference"() -> (w156:refnum<vi>)
        n78 = Not(x=w163) -> (.not. x?=w160:bool)
        n79 = Equal?(x=w162, y=T10."Run Time System" ("Application:Kind")) -> (x = y?=w159:bool)
        n80 = Or(x=w160, y=w159) -> (x .or. y?=w157:bool)
        n81 = Bundle By Name(cluster=w158, "Core.Current VI Reference"=w156, "Core.Close Panel on Exit?"=w157) -> (w165:T13)
        n82 = call <vilib>:"Add State(s) to Queue__JKI_lib_State_Machine.vi"("State(s) in (\"\")"=w167) -> ("States Out"=w166:string)  [unwired: 14 in]
      }
      frame "Error Handler" {
        # "Handle any errors here.\nYou can also output any states to clean-up after errors occur"
        # "Clear error"
        n83 = Unbundle By Name(w173) -> ("Error"=w175:bool)
        n84 = Not(x=w175) -> (.not. x?=w168:bool)
        n85 = Bundle By Name(cluster=w173, "Error"=w168) -> (w174:T13)
        n86 = call-poly <userlib>:"Filter Error Codes__ogtk.vi"("Error In"=w170, "Error Codes to Filter"=i32[] [-200077]) -> ("Error Out"=w169:errorcluster)  [unwired: 7 in, 2 out]
        n87 = case shown="No Error" w169 {
          selector: w169 -> [_ w181]
          tunnel: ["4461: RESET" "Macro: Exit"] -> w172
          frame No Error {
          }
          frame Error {
            w182 = T14 1 items=["no dialog", "OK message", "continue or stop message", "OK message + warnings", "continue/stop + warnings"] ("type of dialog (OK msg:1)")
            # "Unhandled Error -- Display it"
            n88 = call <vilib>:"General Error Handler.vi"("type of dialog (OK msg:1)"=w182, "error in (no error)"=w181) -> ()  [unwired: 9 in, 5 out]
          }
        }
        n89 = call <vilib>:"Add State(s) to Queue__JKI_lib_State_Machine.vi"("State(s) in Front (\"\")"=w172, "State(s) in (\"\")"=w178) -> ("States Out"=w177:string)  [unwired: 13 in]
        "error" <- w170
      }
      frame "Exit" {
        # "Do not put any code in this frame.\n(No errors that occur here will be handled.)"
        n90 = call <vilib>:"Add State(s) to Queue__JKI_lib_State_Machine.vi"("State(s) in (\"\")"=w187) -> ("States Out"=w186:string)  [unwired: 14 in]
      }
      frame "---------- Data ----------" {
        # "Do not put any code in this frame.\n(It is a separator no-op. You can make a copy of this frame to create a new Data frame)"
        n91 = call <vilib>:"Add State(s) to Queue__JKI_lib_State_Machine.vi"("State(s) in (\"\")"=w191) -> ("States Out"=w190:string)  [unwired: 14 in]
      }
      frame "Data: Initialize" {
        w192 = string[] []  # Tasks
        w193 = cluster{"Fs":dbl, "#s":dbl} {"Fs"=204800.0, "#s"=204800.0}  # sampling info
        w194 = waveform(dbl)[] []  # Ouput Signals
        w196 = waveform(dbl)[] []  # Input Signals
        w195 = waveform(dbl)[] []  # REF
        w197 = refnum<k21>[] []  # AO task
        w198 = refnum<k21>[] []  # AI task
        w199 = T15 {"Current VI Reference"=refnum, "Close Panel on Exit?"=FALSE}  # Core
        w201 = FALSE  # Error
        w200 = ""  # Your string data
        # "do not delete - used by framework"
        # "Expand Bundle to add new data elements to shift register data."
        # "Add new data here."
        # "Data names and types of shift register data are defined by this bundle."
        # "Initialize the shift-register data, here.\n(data names are defined by what you wire into the bundle function)"
        n92 = Bundle("Core"=w199, "Error"=w201, "Your string data"=w200, "AI task"=w198, "AO task"=w197, "Input Signals"=w196, "Ouput Signals"=w194, "REF"=w195, "sampling info"=w193, "Tasks"=w192) -> (w203:T13)  [unwired: 1 in]
        n93 = call <vilib>:"Add State(s) to Queue__JKI_lib_State_Machine.vi"("State(s) in (\"\")"=w205) -> ("States Out"=w204:string)  [unwired: 14 in]
      }
      frame "Data: Cleanup" {
        # "Cleanup any data and references, here.\n(this is called automatically, by the Macro: Exit)"
        n94 = Unbundle By Name(w206) -> ("Core.Current VI Reference"=w209:refnum<vi>)
        n95 = Close Reference(reference=w209, error in (no error)=w208) -> (error out=w207:errorcluster)
        n96 = call <vilib>:"Add State(s) to Queue__JKI_lib_State_Machine.vi"("State(s) in (\"\")"=w211) -> ("States Out"=w210:string)  [unwired: 14 in]
      }
      frame "---------- UI ----------" {
        # "Do not put any code in this frame.\n(It is a separator no-op. You can make a copy of this frame to create a new UI frame)"
        n97 = call <vilib>:"Add State(s) to Queue__JKI_lib_State_Machine.vi"("State(s) in (\"\")"=w215) -> ("States Out"=w214:string)  [unwired: 14 in]
      }
      frame "UI: Initialize" {
        w216 = FALSE ("EXIT")
        w220 = waveform(dbl)[][] [] ("History Data")
        # "empty Display charts"
        # "Initialize the User Interface, here.\n(this is called automatically, by the Macro: Init)"
        n98 = local write "error"(errorcluster {"status"=FALSE, "code"=0, "source"=""} ("error out")) -> ()
        n99 = local write "EXIT"(w216) -> ()
        n100 = property on="Display X (or R)" class="WaveformChart (strict)"("History Data"=w220) -> ()  [unwired: 2 in, 2 out]
        n101 = property on="Display Y (or Theta)" class="WaveformChart (strict)"("History Data"=w220) -> ()  [unwired: 2 in, 2 out]
        n102 = local write "RESET"(w216) -> ()
        n103 = local write "Bug"(w216) -> ()
        n104 = call <vilib>:"Add State(s) to Queue__JKI_lib_State_Machine.vi"("State(s) in (\"\")"=w222) -> ("States Out"=w221:string)  [unwired: 14 in]
      }
      frame "UI: Cursor Set" {
        # "Argument"
        # "Set and Unset Cursor Busy.\n(Usage: \"UI: Cursor Set >> Busy|Idle\")"
        n105 = case shown="\"Busy\"" w224 {
          tunnel: w226 -> [w230 w232]
          tunnel: [w229 w231] -> w225
          frame "Idle", Default {
            n106 = call <vilib>:"Unset Busy.vi"("error in (no error)"=w230) -> ("error out"=w229:errorcluster)  [unwired: 10 in]
          }
          frame "Busy" {
            n107 = call <vilib>:"Set Busy.vi"("error in (no error)"=w232) -> ("error out"=w231:errorcluster)  [unwired: 9 in, 1 out]
          }
        }
        n108 = call <vilib>:"Add State(s) to Queue__JKI_lib_State_Machine.vi"("State(s) in (\"\")"=w228) -> ("States Out"=w227:string)  [unwired: 14 in]
      }
      frame "UI: Front Panel State" {
        # "Argument"
        # "Set Front Panel Open or Closed\n(Usage: \"UI: Front Panel State >> Open|Close\")"
        n109 = Unbundle By Name(w234) -> ("Core.Current VI Reference"=w236:refnum<vi>)
        n110 = case shown="\"Open\", Default" w235 {
          tunnel: w237 -> [w243 w256]
          tunnel: [w245 w257] -> w233
          tunnel: w236 -> [w244 w254]
          frame "Open", Default {
            n111 = property class="VI"(reference=w244, error in=w243) -> (reference out=w241:refnum<vi>, error out=w242:errorcluster, "Front Panel.Open"=w240:bool)
            n112 = case shown="True" w240 {
              tunnel: [w248 w251] -> w245
              tunnel: w242 -> [w247 w251]
              tunnel: w241 -> [w246 _]
              frame False {
                n113 = invoke class="VI" method="FP.Open"(reference=w246, error in=w247, "Activate"=TRUE, "State"=T11."Standard") -> (error out=w248:errorcluster)  [unwired: 1 in, 4 out]
              }
              frame True {
              }
            }
          }
          frame "Close" {
            n114 = property class="VI"(reference=w254, error in=w256) -> (reference out=w253:refnum<vi>, error out=w255:errorcluster, "Front Panel.Open"=w252:bool)
            n115 = case shown="True" w252 {
              tunnel: [w258 w261] -> w257
              tunnel: w255 -> [w258 w260]
              tunnel: w253 -> [_ w259]
              frame False {
              }
              frame True {
                n116 = invoke class="VI" method="FP.Close"(reference=w259, error in=w260) -> (error out=w261:errorcluster)  [unwired: 1 in, 2 out]
              }
            }
          }
        }
        n117 = call <vilib>:"Add State(s) to Queue__JKI_lib_State_Machine.vi"("State(s) in (\"\")"=w239) -> ("States Out"=w238:string)  [unwired: 14 in]
      }
      frame "---------- Macro ----------" {
        # "Do not put any code in this frame.\n(It is a separator no-op. You can make a copy of this frame to create a new Macro frame)"
        n118 = call <vilib>:"Add State(s) to Queue__JKI_lib_State_Machine.vi"("State(s) in (\"\")"=w265) -> ("States Out"=w264:string)  [unwired: 14 in]
      }
      frame "Macro: Initialize" {
        w267 = "Data: Initialize\nInitialize Core Data\nUI: Initialize\nUI: Front Panel State >> Open\n#4461: Setup\n#4461: Create Tasks"  # Data: Initialize Initialize Core Data UI: Initialize UI: Front Panel State >> Open #4461: Setup #4461: Create Tasks
        # "Initialization Macro\n(This is called once, when the VI starts)"
        n119 = call <vilib>:"Add State(s) to Queue__JKI_lib_State_Machine.vi"("State(s) in Front (\"\")"=w267, "State(s) in (\"\")"=w270) -> ("States Out"=w269:string)  [unwired: 13 in]
      }
      frame "Macro: Exit" {
        w272 = FALSE ("EXIT")
        # "Exit Macro\n(This is called once, when the VI exits)"
        n120 = Unbundle By Name(w271) -> ("Core.Close Panel on Exit?"=w278:bool)
        n121 = local write "EXIT"(w272) -> ()
        n122 = local write "RESET"(w272) -> ()
        n123 = Select(t="UI: Front Panel State >> Close", s=w278, f="") -> (s? t:f=w275:string)
        n124 = call <vilib>:"Add State(s) to Queue__JKI_lib_State_Machine.vi"("State(s) in (\"\")"=w275, "State(s) at Back (\"\")"="Data: Cleanup\nExit") -> ("States Out"=w273:string)  [unwired: 13 in]
        n125 = call <vilib>:"Add State(s) to Queue__JKI_lib_State_Machine.vi"("State(s) in Front (\"\")"=w273, "State(s) in (\"\")"=w281) -> ("States Out"=w280:string)  [unwired: 13 in]
      }
      frame "---------- 4461----------" {
        n126 = call <vilib>:"Add State(s) to Queue__JKI_lib_State_Machine.vi"("State(s) in (\"\")"=w285) -> ("States Out"=w284:string)  [unwired: 14 in]
      }
      frame "4461: INI" {
        n127 = case shown="True" "save config" {
          tunnel: "Instrument" -> [w303 w307]
          tunnel: w289 -> [w301 w306]
          tunnel: [w300 w305] -> w288
          tunnel: "load config" -> [_ w304]
          frame True {
            n128 = local read "AI Configuration"() -> (w297:T7)
            n129 = local read "AO Configuration"() -> (w298:T6)
            n130 = local read "DAQ Type"() -> (w299:enum16{"None", "USB 4431", "PXI 446x"})
            n131 = local read "Amplifiers"() -> (w296:enum16{"None", "Krohn Hite", "Femto"})
            n132 = call "config.vi"("Function"=enum16{"write", "read"}."write", "Error In"=w301, "Instrument"=w303, "Amplifiers"=w296, "DAQ Type"=w299, "AO Configuration"=w298, "AI Configuration"=w297) -> ("Error Out"=w300:errorcluster)  [unwired: 4 out]
            n133 = local write "save config"(FALSE ("save config")) -> ()
          }
          frame False {
            n134 = case shown="True" w304 {
              tunnel: w307 -> [_ w313]
              tunnel: w306 -> [w308 w311]
              tunnel: [w308 w310] -> w305
              frame False {
              }
              frame True {
                n135 = local write "load config"(FALSE ("load config")) -> ()
                n136 = call "config.vi"("Function"=enum16{"write", "read"}."read", "Error In"=w311, "Instrument"=w313) -> ("Amplifiers"=w316:enum16{"None", "Krohn Hite", "Femto"}, "DAQ Type"=w317:enum16{"None", "USB 4431", "PXI 446x"}, "AO Configuration 2"=w314:T6, "AI Configuration 2"=w315:T7, "Error Out"=w310:errorcluster)  [unwired: 4 in]
                n137 = local write "AI Configuration"(w315) -> ()
                n138 = local write "AO Configuration"(w314) -> ()
                n139 = local write "DAQ Type"(w317) -> ()
                n140 = local write "Amplifiers"(w316) -> ()
              }
            }
          }
        }
        n141 = call <vilib>:"Add State(s) to Queue__JKI_lib_State_Machine.vi"("State(s) in (\"\")"=w292, "State(s) at Back (\"\")"="4461: RESET" ("State(s) at Back (\"\")")) -> ("States Out"=w293:string)  [unwired: 13 in]
      }
      frame "4461: SETUP" {
        n142 = local read "Channels: AO"() -> (w320:T8)
        n143 = Unbundle By Name(w332) -> ("sampling info"=w333:cluster{"Fs":dbl, "#s":dbl})
        n144 = case shown="\"None\"" "DAQ Type" {
          frame "USB 4431", Default {
          }
          frame "PXI 446x" {
          }
          frame "None" {
            n145 = local write "Amplifiers"(enum16{"None", "Krohn Hite", "Femto"}."None" ("Amplifiers")) -> ()
          }
        }
        n146 = case shown="\"None\"" "DAQ Type" {
          tunnel: [u32 0 u32 0 u32 16448250] -> w328
          tunnel: [u32 6618880 u32 6618880 u32 16711680] -> w327
          frame "USB 4431" {
          }
          frame "PXI 446x" {
          }
          frame "None" {
          }
        }
        n147 = Unbundle By Name(w320) -> ("AO f (Hz)"=w318:dbl[])
        n148 = Index Array(array=w318) -> (element=w322:dbl)  [unwired: 1 in]
        n149 = property on="DAQ mode string" class="Str"("Text.BG Color"=w327, "Text.FG Color"=w328) -> ()  [unwired: 2 in, 2 out]
        n150 = property on="DAQ Type" class="Enum (strict)"() -> ("RingText.Text"=→"DAQ mode string":string)  [unwired: 2 in, 2 out]
        n151 = Bundle(cluster=cluster{"Fs":i32, "#s":i32} {"Fs"=204000, "#s"=34} ("sampling info"), "Fs"="Fs", "#s"="#s") -> (w323:cluster{"Fs":i32, "#s":i32})
        "sampling info" <- w323
        n152 = case shown="True" "auto size" {
          tunnel: w333 -> [_ w358]
          tunnel: [w344 w359] -> w331
          tunnel: w322 -> [_ w345]
          tunnel: "DAQ Type" -> [_ w352]
          tunnel: w323 -> [w344 _]
          frame False {
          }
          frame True {
            n153 = case shown="\"PXI 446x\"" w352 {
              tunnel: [102400.0 ("upper limit") 204800.0 ("upper limit") 204800.0 ("upper limit")] -> w346
              frame "USB 4431", Default {
              }
              frame "PXI 446x" {
              }
              frame "None" {
              }
            }
            n154 = Multiply(x="frequency multiplier", y=w345) -> (x*y=w357:dbl)
            n155 = In Range and Coerce(upper limit=w346, x=w357, lower limit=1000.0) -> (coerced(x)=w355:dbl)  [unwired: 1 out]
            n156 = call "Fs and Ns for integer periods.vi"("f_integer"=w345, "Fs"=w355) -> ("#s_integer"=w348:dbl, "Fs_integer"=w350:dbl)  [unwired: 8 in]
            n157 = In Range and Coerce(upper limit=w346, x=w348, lower limit=128.0) -> (coerced(x)=w347:dbl)  [unwired: 1 out]
            n158 = In Range and Coerce(upper limit=w346, x=w350, lower limit=1000.0) -> (coerced(x)=w351:dbl)  [unwired: 1 out]
            n159 = local write "#s"(w347) -> ()
            n160 = Bundle By Name(cluster=w358, "Fs"=w351, "#s"=w347) -> (w359:cluster{"Fs":dbl, "#s":dbl})
            n161 = local write "Fs"(w351) -> ()
          }
        }
        n162 = Bundle By Name(cluster=w332, "sampling info"=w331) -> (w330:T13)
        n163 = call <vilib>:"Add State(s) to Queue__JKI_lib_State_Machine.vi"("State(s) in (\"\")"=w336) -> ("States Out"=w335:string)  [unwired: 14 in]
      }
      frame "4461: CREATE TASKS" {
        w370 = 10178 items=["Finite Samples"=10178, "Continuous Samples"=10123] ("sample mode")
        w369 = 10123 items=["Finite Samples"=10178, "Continuous Samples"=10123] ("sample mode")
        n164 = local read "AO Configuration"() -> (w374:T6)
        n165 = local read "Channels: Lockin"() -> (w367:T9)
        n166 = local read "AI Configuration"() -> (w376:T7)
        n167 = local read "AI Buffer Size (S)"() -> (w381:i32)
        n168 = Unbundle By Name(w371) -> ("sampling info"=w372:cluster{"Fs":dbl, "#s":dbl})
        n169 = local read "Channels: AO"() -> (w382:T8)
        n170 = local read "DAQ Type"() -> (w366:enum16{"None", "USB 4431", "PXI 446x"})
        n171 = local read "IV Curve Mode"() -> (w363:bool)
        n172 = Equal?(x=w366, y=enum16{"None", "USB 4431", "PXI 446x"}."None" ("DAQ Type")) -> (x = y?=w364:bool)
        n173 = Select(t=w370, s=w363, f=w369) -> (s? t:f=w368:i32)
        n174 = case shown="True" w364 {
          tunnel: w376 -> [w396 _]
          tunnel: w374 -> [w395 _]
          tunnel: [w394 w415] -> w380
          tunnel: w372 -> [w393 w412]
          tunnel: [w392 w415] -> w379
          tunnel: w381 -> [w391 _]
          tunnel: [w390 dbl[] [] ("phase log")] -> w375
          tunnel: w382 -> [w389 w413]
          tunnel: w377 -> [w388 w418]
          tunnel: [w387 w417] -> w373
          tunnel: w368 -> [w386 _]
          tunnel: w367 -> [w385 w414]
          tunnel: w363 -> [_ w411]
          frame False {
            n175 = disable-structure shown="Default" {
              disable-tunnel: w396 -> [w408 _]
              disable-tunnel: w395 -> [w407 _]
              disable-tunnel: [w406 _] -> w394
              disable-tunnel: w393 -> [w403 _]
              disable-tunnel: [w405 _] -> w392
              disable-tunnel: w391 -> [w401 _]
              disable-tunnel: [w402 _] -> w390
              disable-tunnel: w389 -> [w404 _]
              disable-tunnel: w388 -> [w400 _]
              disable-tunnel: [w399 _] -> w387
              disable-tunnel: w386 -> [w398 _]
              disable-tunnel: w385 -> [w397 _]
              frame condition #0 (active) {
                n176 = call "4461 - Create IO Channels Parallel Uneven.vi"("sample mode"=w398, "Channels: Lockin"=w397, "error in"=w400, "AI Buffer Size (S)"=w401, "sampling info"=w403, "AO"=w404, "AO Configuration"=w407, "AI Configuration"=w408) -> ("AO Task"=w405:refnum<k21>[], "AI task"=w406:refnum<k21>[], "error out"=w399:errorcluster, "phase log"=w402:dbl[])
              }
              frame condition #1 {
              }
            }
          }
          frame True {
            w415 = refnum<k21>[] [] ("AI task")
            # "simulate mode"
            n177 = Not(x=w411) -> (.not. x?=w410:bool)
            n178 = Initialize Array(1.0 ("element"), 8 ("dimension size")) -> (w409:dbl[])
            n179 = call "4461 - Create AO waveforms.vi"("sampling info"=w412, "reset signal"=w410, "AO"=w413) -> ()  [unwired: 5 in, 4 out]
            n180 = call "4461 - Create Reference Waveforms.vi"("sampling info"=w412, "reset signal"=w410, "Lockin"=w414) -> ()  [unwired: 5 in, 4 out]
            n181 = call <userlib>:"FGV - KH Gain.vi"("error in"=w418, "Function"=enum16{"write", "read"}."write", "Array"=w409) -> ("error out"=w417:errorcluster)  [unwired: 3 in, 1 out]
            n182 = local write "Gain"(w409) -> ()
          }
        }
        n183 = local write "phase log"(w375) -> ()
        n184 = Bundle By Name(cluster=w371, "AI task"=w380, "AO task"=w379) -> (w378:T13)
        n185 = call <vilib>:"Add State(s) to Queue__JKI_lib_State_Machine.vi"("State(s) in (\"\")"=w384) -> ("States Out"=w383:string)  [unwired: 14 in]
      }
      frame "4461: READ WRITE" {
        n186 = Unbundle By Name(w452) -> ("sampling info"=w435:cluster{"Fs":dbl, "#s":dbl}, "AI task"=w451:refnum<k21>[])
        n187 = local read "IV Curve Mode"() -> (w422:bool)
        n188 = local read "..........reset signal"() -> (w424:bool)
        n189 = local read "....measure offset"() -> (w450:bool)
        n190 = local read "Channels: AO"() -> (w444:T8)
        n191 = Unbundle By Name(w444) -> ("AO amp (V)"=w441:dbl[])
        n192 = Array Size(array=w441) -> (size(s)=w442:i32)
        n193 = Initialize Array(0.0 ("element"), w442) -> (w439:dbl[])
        n194 = local read "Channels: Lockin"() -> (w448:T9)
        n195 = Bundle By Name(cluster=w444, "AO amp (V)"=w439) -> (w443:T8)
        n196 = Get Date/Time In Seconds() -> (seconds since 1Jan1904=w432:timestamp)
        n197 = Select(t=FALSE, s=w422, f=w424) -> ()  [unwired: 1 out]
        n198 = Format Date/Time String(time format string (%c)="%H:%M:%S%1u   %Y-%m-%d", seconds (now)=w432) -> (date/time string=→"time and date":string)  [unwired: 1 in]
        n199 = Select(t=w443, s=w450, f=w444) -> (s? t:f=w449:T8)
        n200 = Or(x=w422, y=w424) -> (x .or. y?=w423:bool)
        n201 = call "4461 - Create AO waveforms.vi"("error in (no error)"=w462, "sampling info"=w435, "reset signal"=w423, "AO"=w449) -> ("error out"=w447:errorcluster, "phase out"=w445:dbl[], "AO Array"=w446:waveform(dbl)[])  [unwired: 4 in, 1 out]
        n202 = call "4461 - Create Reference Waveforms.vi"("error in (no error)"=w462, "sampling info"=w435, "reset signal"=w423, "Lockin"=w448) -> ("error out"=w454:errorcluster, "AO Array"=w438:waveform(dbl)[])  [unwired: 4 in, 2 out]
        n203 = local read "DAQ Type"() -> (w434:enum16{"None", "USB 4431", "PXI 446x"})
        n204 = call-poly <userlib>:"Empty Array__ogtk.vi"("Array"=w451) -> ("Empty Array?"=w427:bool)  [unwired: 8 in]
        n205 = local write "phase log"(w445) -> ()
        n206 = Equal?(x=w434, y=enum16{"None", "USB 4431", "PXI 446x"}."None" ("DAQ Type")) -> (x = y?=w433:bool)
        n207 = Or(x=w427, y=w433) -> (x .or. y?=w428:bool)
        n208 = case shown="False" w428 {
          tunnel: [w482 w496] -> w436
          tunnel: w446 -> [w476 w494]
          tunnel: w435 -> [w477 w493]
          tunnel: w452 -> [w479 _]
          tunnel: w447 -> [w478 w495]
          tunnel: [w480 w495] -> w461
          tunnel: [w475 w494] -> w437
          tunnel: w422 -> [w473 _]
          frame False {
            n209 = Unbundle By Name(w479) -> ("AI task"=w481:refnum<k21>[], "AO task"=w474:refnum<k21>[])
            n210 = disable-structure shown="Default" {
              disable-tunnel: [w484 _] -> w482
              disable-tunnel: w476 -> [w485 w491]
              disable-tunnel: w477 -> [w486 _]
              disable-tunnel: w481 -> [w488 _]
              disable-tunnel: w478 -> [w490 _]
              disable-tunnel: [w489 _] -> w480
              disable-tunnel: [w485 w491] -> w475
              disable-tunnel: w474 -> [w487 _]
              disable-tunnel: w473 -> [w483 _]
              frame condition #0 (active) {
                n211 = call "4461 - AI AND AI - Read AND Write Uneven.vi"("IV Curve Mode"=w483, "AO Array"=w485, "error in (no error)"=w490, "sampling info"=w486, "AO Task"=w487, "AI task"=w488) -> ("error out"=w489:errorcluster, "Input Signals"=w484:waveform(dbl)[])  [unwired: 4 in]
              }
              frame condition #1 {
              }
            }
            n212 = property on="DAQ mode string" class="Str"("Text.BG Color"=u32 6618880) -> ()  [unwired: 2 in, 2 out]
          }
          frame True {
            n213 = call "4461 Sim - Noise.vi"("data"=w494, "sampling info"=w493) -> ("Data"=w496:waveform(dbl)[])  [unwired: 5 in]
            n214 = local write "DAQ Type"(enum16{"None", "USB 4431", "PXI 446x"}."None" ("DAQ Type")) -> ()
          }
        }
        n215 = case shown="True" w427 {
          frame False {
          }
          frame True {
            # "flash colors to alert user"
            n216 = property on="DAQ mode string" class="Str"() -> ("Text.BG Color"=w468:u32)  [unwired: 2 in, 2 out]
            n217 = Equal?(x=w468, y=u32 16711680) -> (x = y?=w467:bool)
            n218 = case shown="False" w467 {
              tunnel: [u32 16711680 u32 16448250] -> w466
              frame False {
              }
              frame True {
              }
            }
            n219 = property on="DAQ mode string" class="Str"("Text.BG Color"=w466) -> ()  [unwired: 2 in, 2 out]
          }
        }
        n220 = Index Array(array=w436) -> (element=w459:waveform(dbl))  [unwired: 1 in]
        n221 = local write "time since trigger"(0.0 ("time since trigger")) -> ()
        n222 = Unbundle By Name(w459) -> ("Y"=w458:dbl[])
        n223 = Bundle By Name(cluster=w452, "Input Signals"=w436, "Ouput Signals"=w437, "REF"=w438) -> (w463:T13)
        n224 = call-poly <userlib>:"Empty Array__ogtk.vi"("Array"=w458) -> ("Empty Array?"=w456:bool)  [unwired: 8 in]
        n225 = Merge Errors(w461, w454) -> (w460:errorcluster)
        n226 = Select(t="4461: RESET" ("State(s) at Back (\"\")"), s=w456, f="" ("State(s) at Back (\"\")")) -> (s? t:f=w425:string)
        n227 = call <vilib>:"Add State(s) to Queue__JKI_lib_State_Machine.vi"("State(s) in Front (\"\")"=w425, "State(s) in (\"\")"=w465) -> ("States Out"=w464:string)  [unwired: 13 in]
      }
      frame "4461: FILTER" {
        w499 = TRUE ("averaging")
        n228 = Unbundle By Name(w501) -> ("Ouput Signals"=w498:waveform(dbl)[], "Input Signals"=w520:waveform(dbl)[], "REF"=w510:waveform(dbl)[])
        n229 = local read "decimating factor"() -> (w503:i32)
        n230 = call "decimate_waveforms.vi"("decimating factor"=w503, "averaging"=w499, "error in (no error)"=w515, "Input Signal"=w498) -> ("error out"=w514:errorcluster, "Decimated Waveforms"=w497:waveform(dbl)[])  [unwired: 6 in]
        n231 = call "decimate_waveforms.vi"("decimating factor"=w503, "averaging"=w499, "error in (no error)"=w515, "Input Signal"=w520) -> ("error out"=w517:errorcluster, "Decimated Waveforms"=w508:waveform(dbl)[])  [unwired: 6 in]
        n232 = call "decimate_waveforms.vi"("decimating factor"=w503, "averaging"=w499, "error in (no error)"=w515, "Input Signal"=w510) -> ("error out"=w516:errorcluster, "Decimated Waveforms"=w502:waveform(dbl)[])  [unwired: 6 in]
        n233 = local read "offsets"() -> (w521:dbl[])
        n234 = Subtract(x=w508, y=w521) -> (x-y=w507:waveform(dbl)[])
        n235 = Merge Errors(w514, w517, w516) -> (w512:errorcluster)
        n236 = case shown="False" "60 Hz prefilter" {
          tunnel: w507 -> [w529 w531]
          tunnel: [w529 w530] -> w506
          frame False {
          }
          frame True {
            n237 = call "Prefilter_60Hz_Notch.vi"("Array"=w531) -> ("Array 2"=w530:waveform(dbl)[])  [unwired: 10 in]
          }
        }
        n238 = local read "............zero offset"() -> (w511:bool)
        n239 = local read "....measure offset"() -> (w513:bool)
        n240 = Index Array(array=w502) -> (element=w519:waveform(dbl))  [unwired: 1 in]
        n241 = case shown="False" "LP prefilter" {
          tunnel: w506 -> [w525 w528]
          tunnel: [w525 w527] -> w505
          tunnel: "LP cutoff (Hz)" -> [_ w526]
          frame False {
          }
          frame True {
            n242 = call "Prefilter_LP.vi"("high cutoff freq [Hz]"=w526, "Array"=w528) -> ("Array 2"=w527:waveform(dbl)[])  [unwired: 9 in]
          }
        }
        n243 = Unbundle By Name(w519) -> ("dt"=w518:dbl)
        n244 = local write "dt"(w518) -> ()
        n245 = case shown="False" w513 {
          tunnel: w501 -> [w535 w540]
          frame False {
            n246 = Unbundle By Name(w535) -> ("Input Signals"=w534:waveform(dbl)[])
            n247 = for {
              tunnel: w534 -> [w537] mode=indexing
              tunnel: [w536] -> w533 mode=indexing
              n248 = call-poly <vilib>:"Mean.vi"("X"=w537) -> ("mean"=w536:dbl)  [unwired: 1 out]
            }
            n249 = local write "mean"(w533) -> ()
          }
          frame True {
            n250 = Unbundle By Name(w540) -> ("Input Signals"=w539:waveform(dbl)[])
            n251 = for {
              tunnel: w539 -> [w542] mode=indexing
              tunnel: [w541] -> w538 mode=indexing
              n252 = call-poly <vilib>:"Mean.vi"("X"=w542) -> ("mean"=w541:dbl)  [unwired: 1 out]
            }
            n253 = local write "offsets"(w538) -> ()
            n254 = local write "mean"(w538) -> ()
          }
        }
        n255 = case shown="False" w511 {
          frame False {
          }
          frame True {
            n256 = local write "offsets"(dbl[] [0.0, 0.0, 0.0, 0.0, 0.0, 0.0, 0.0, 0.0] ("offsets")) -> ()
          }
        }
        n257 = Bundle By Name(cluster=w501, "Ouput Signals"=w497, "Input Signals"=w505, "REF"=w502) -> (w522:T13)
        n258 = call <vilib>:"Add State(s) to Queue__JKI_lib_State_Machine.vi"("State(s) in (\"\")"=w524) -> ("States Out"=w523:string)  [unwired: 14 in]
      }
      frame "4461: PHASE" {
        n259 = local read "Results\n(X, Y, R, Theta, mean)"() -> (w554:dbl[][])
        n260 = local read "autophase?\n(experimental)"() -> (w553:bool)
        n261 = local read "phase log"() -> (w555:dbl[])
        n262 = local read "Channels: Lockin"() -> (w551:T9)
        n263 = local read "Channels: AO"() -> (w550:T8)
        n264 = call "lockin - Set all f same.vi"("all  frequencies same?"="............all  f same", "Lockin"=w551, "AO"=w550) -> ("Lockin 2"=w548:T9, "AO 2"=w547:T8)  [unwired: 7 in]
        n265 = call "lockin - Set REF phase equals zero.vi"("reset REF phi to zero"="...............reset REF", "Channels: Lockin"=w548, "Channels: AO"=w547) -> ("Channels: Lockin 2"=w543:T9, "Channels: AO 2"=w549:T8)  [unwired: 7 in]
        n266 = case shown="True" w553 {
          tunnel: w555 -> [_ w564]
          tunnel: w554 -> [_ w563]
          tunnel: w543 -> [w559 w561]
          tunnel: [w559 w560] -> w544
          frame False {
          }
          frame True {
            # "do this for EACH lockin...\n- replace PID array with PID SV\n-  advance \"results\" by 8?\n- this should go BEFORE REF\nwaveform is generated"
            n267 = Index Array(array=w563, index (col)=3 ("index (row)")) -> (element=w566:dbl[])  [unwired: 1 in]
            n268 = call "Simple PID Array.vi"("D"="D", "I"="I", "P"="P", "process variable"=w566) -> ("output value"=w570:dbl[])  [unwired: 7 in]
            n269 = Subtract(x=w564, y=w570) -> (x-y=w562:dbl[])
            n270 = Bundle By Name(cluster=w561, "REF phi (deg)"=w562) -> (w560:T9)
          }
        }
        n271 = local write "Channels: AO"(w549) -> ()
        n272 = local write "Channels: Lockin"(w544) -> ()
        n273 = call <vilib>:"Add State(s) to Queue__JKI_lib_State_Machine.vi"("State(s) in (\"\")"=w558) -> ("States Out"=w557:string)  [unwired: 14 in]
      }
      frame "4461: LOCKIN" {
        (unwired) 0
        # "Display stuff and lockin calculations"
        n274 = Unbundle By Name(w619) -> ("Ouput Signals"=w575:waveform(dbl)[], "Input Signals"=w593:waveform(dbl)[], "REF"=w574:waveform(dbl)[], "sampling info"=w583:cluster{"Fs":dbl, "#s":dbl})
        n275 = local read "TC (s)"() -> (w617:dbl)
        n276 = local read "mean"() -> (w611:dbl[])
        n277 = local read "order"() -> (w616:i32)
        n278 = local read "Gain"() -> (w581:dbl[])
        n279 = local read "Gain"() -> (w580:dbl[])
        n280 = Select(t="applied signals (V)" ("Y Scale.Name Label.Text"), s="Output signals?", f="REF signal (arb)" ("Y Scale.Name Label.Text")) -> (s? t:f=w582:string)
        n281 = Select(t=w575, s="Output signals?", f=w574) -> (s? t:f=w589:waveform(dbl)[])
        n282 = Divide(x=w593, y=w580) -> (x/y=w578:waveform(dbl)[])
        n283 = property on="Reference Graph" class="WFGraph (strict)"("YScale.NameLbl.Text"=w582) -> ()  [unwired: 2 in, 2 out]
        n284 = Divide(x=w611, y=w581) -> (x/y=w610:dbl[])
        n285 = call "Display n or dt.vi"("Display n?"="Display n?", "Input Waveforms"=w593) -> ("Output Waveforms"=w597:waveform(dbl)[])  [unwired: 9 in]
        n286 = call "Display n or dt.vi"("Display n?"="Display n?", "Input Waveforms"=w589) -> ("Output Waveforms"=w595:waveform(dbl)[])  [unwired: 9 in]
        n287 = call "decimate_waveforms.vi"("decimating factor"="decimate graph", "averaging"=FALSE, "Input Signal"=w595) -> ("Decimated Waveforms"=→"Reference Graph":waveform(dbl)[])  [unwired: 7 in, 1 out]
        n288 = call "decimate_waveforms.vi"("decimating factor"="decimate graph", "averaging"=FALSE, "Input Signal"=w597) -> ("Decimated Waveforms"=→"Signals Graph":waveform(dbl)[])  [unwired: 7 in, 1 out]
        n289 = call "4461 - Lockin Engine.vi"("order"=w616, "TC (s)"=w617, "sampling info"=w583, "Reference In"=w574, "Signal in"=w578) -> ("filter fC (Hz)"=w587:dbl, "Results (X,Y,R,Theta)"=w613:dbl[][])  [unwired: 5 in]
        n290 = Transpose 2D Array(2D array=w613) -> (transposed array=w606:dbl[][])
        n291 = Build Array (concatenate)(w606, w610) -> (w612:dbl[][])
        n292 = Index Array(array=w578) -> (element=w590:waveform(dbl))  [unwired: 1 in]
        n293 = call "FGV - Signals - Output.vi"("Function"=enum16{"write", "read"}."write", "input signal"=w575) -> ()  [unwired: 4 in, 2 out]
        n294 = call "FGV - Signals - Input.vi"("Function"=enum16{"write", "read"}."write", "input signal"=w578) -> ()  [unwired: 4 in, 2 out]
        n295 = local read "Channel"() -> (w588:dbl)
        n296 = local write "filter fC (Hz)"(w587) -> ()
        n297 = local read "Display"() -> (w615:enum16{"X and Y", "R and Theta"})
        n298 = Transpose 2D Array(2D array=w612) -> (transposed array=w594:dbl[][])
        "Results\n(X, Y, R, Theta, mean)" <- w594
        n299 = Unbundle By Name(w590) -> ("t0"=w577:timestamp)
        n300 = local read "Tab Control 2"() -> (w609:T1)
        n301 = call "format display.vi"("Channel"=w588, "Display"=w615, "Results (X,Y,R,Theta)"=w613, "t0"=w577) -> ("X/R"=→"X or R":dbl, "Array 2"=→"XY Graph":cluster{dbl[], dbl[]}[], "Y/Theta Array"=→"Display Y (or Theta)":waveform(dbl)[], "X/R Array"=→"Display X (or R)":waveform(dbl)[], "Y/R"=→"Y or Theta":dbl)  [unwired: 3 in]
        n302 = call "FGV - Lockin Results.vi"("Function"=enum16{"write", "read"}."write", "Input Signals"=w594) -> ()  [unwired: 4 in, 2 out]
        n303 = Equal?(x=w609, y=T12."PS" ("Tab Control 2")) -> (x = y?=w576:bool)
        n304 = Select(t="4461: FFT" ("State(s) at Back (\"\")"), s=w576, f="" ("State(s) at Back (\"\")")) -> (s? t:f=w572:string)
        n305 = call <vilib>:"Add State(s) to Queue__JKI_lib_State_Machine.vi"("State(s) in (\"\")"=w621, "State(s) at Back (\"\")"=w572) -> ("States Out"=w618:string)  [unwired: 13 in]
      }
      frame "4461: FFT" {
        n306 = Unbundle By Name(w642) -> ("Input Signals"=w624:waveform(dbl)[])
        n307 = local read "Gain"() -> (w640:dbl[])
        n308 = Divide(x=w624, y=w640) -> (x/y=w631:waveform(dbl)[])
        n309 = call-poly <vilib>:"FFT Power Spectrum and PSD.vi"("window parameter"="window parameter", "export mode"="export mode", "averaging parameters"="averaging parameters", "restart averaging (F)"="restart averaging (F)", "dB On (F)"=TRUE, "window"="window", "time signals"=w631) -> ("averages completed"=→"averages\ncompleted":dbl, "averaging done"=→"averaging done":bool, "Power Spectrum / PSD"=w622:cluster{"f0":dbl, "df":dbl, "magnitude":dbl[]}[])  [unwired: 1 in, 1 out]
        "PS dB" <- w622
        n310 = for {
          tunnel: w622 -> [w662] mode=indexing
          tunnel: [w657] -> w623 mode=indexing
          n311 = Unbundle By Name(w662) -> ("df"=w664:dbl, "magnitude"=w663:dbl[])  [unwired: 1 out]
          n312 = Bundle By Name("dt"=w664, "Y"=w663) -> (w661:waveform(dbl))  [unwired: 1 in]
          n313 = call-poly <vilib>:"Waveform to XY Pairs.vi"("waveform in"=w661) -> ("XY pairs"=w660:cluster{"x":timestamp, "y":dbl}[])  [unwired: 8 in, 2 out]
          n314 = for {
            tunnel: w660 -> [w668] mode=indexing
            tunnel: [w666] -> w658 mode=indexing
            tunnel: [w665] -> w659 mode=indexing
            n315 = Unbundle(w668) -> ("x"=w667:timestamp, "y"=w666:dbl)
            n316 = To Double Precision Float(number=w667) -> (double precision float=w665:dbl)
          }
          n317 = Bundle(w659, w658) -> (w657:cluster{dbl[], dbl[]})  [unwired: 1 in]
        }
        n318 = property on="PS dB" class="WFGraph (strict)"("Active Cursor"=u32 1) -> ("Cursor.Cursor X"=w636:dbl)  [unwired: 2 in, 2 out]
        n319 = property on="PS dB" class="WFGraph (strict)"("Active Cursor"=u32 0) -> ("Cursor.Cursor X"=w637:dbl)  [unwired: 2 in, 2 out]
        n320 = Build Array(w637, w636) -> (w635:dbl[])
        n321 = for {
          tunnel: w623 -> [w656] mode=indexing
          tunnel: w635 -> [w655]
          tunnel: [w647] -> w634 mode=indexing
          n322 = Array Max & Min(array=w655) -> (max value=w654:dbl, min value=w652:dbl)  [unwired: 2 out]
          n323 = Unbundle(w656) -> (w653:dbl[], w651:dbl[])
          n324 = Threshold 1D Array(2:w654, 3:w653) -> (0:w650:dbl)  [unwired: 1 in]
          n325 = Threshold 1D Array(2:w652, 3:w653) -> (0:w649:dbl)  [unwired: 1 in]
          n326 = Subtract(x=w650, y=w649) -> (x-y=w648:dbl)
          n327 = Array Subset(array=w651, index=w649, length=w648) -> (w646:dbl[])
          n328 = Add Array Elements(numeric array=w646) -> (sum=w647:dbl)
        }
        n329 = Build Array(w634) -> (→"PS Chart":dbl[][])
        n330 = call <vilib>:"Add State(s) to Queue__JKI_lib_State_Machine.vi"("State(s) in (\"\")"=w645) -> ("States Out"=w643:string)  [unwired: 14 in]
      }
      frame "4461: SAVE" {
        w671 = "FFT" ("filename")
        w670 = "signal" ("filename")
        # "Wait for Trigger signal from other VI"
        n331 = local read "PS dB"() -> (w687:cluster{"f0":dbl, "df":dbl, "magnitude":dbl[]}[])
        n332 = Get Date/Time In Seconds() -> (seconds since 1Jan1904=w678:timestamp)
        n333 = local read "Path"() -> (w669:path)
        n334 = for {
          tunnel: w687 -> [w707] mode=indexing
          tunnel: [w702] -> w682 mode=indexing
          n335 = Unbundle By Name(w707) -> ("df"=w709:dbl, "magnitude"=w708:dbl[])  [unwired: 1 out]
          n336 = Bundle By Name("dt"=w709, "Y"=w708) -> (w706:waveform(dbl))  [unwired: 1 in]
          n337 = call-poly <vilib>:"Waveform to XY Pairs.vi"("waveform in"=w706) -> ("XY pairs"=w705:cluster{"x":timestamp, "y":dbl}[])  [unwired: 8 in, 2 out]
          n338 = for {
            tunnel: w705 -> [w713] mode=indexing
            tunnel: [w711] -> w703 mode=indexing
            tunnel: [w710] -> w704 mode=indexing
            n339 = Unbundle(w713) -> ("x"=w712:timestamp, "y"=w711:dbl)
            n340 = To Double Precision Float(number=w712) -> (double precision float=w710:dbl)
          }
          n341 = Bundle(w704, w703) -> (w702:cluster{dbl[], dbl[]})  [unwired: 1 in]
        }
        n342 = call "FGV - Signals - Input.vi"("error in"=w679, "Function"=enum16{"write", "read"}."read") -> ("error out"=w680:errorcluster, "input signal"=w686:waveform(dbl)[])  [unwired: 4 in]
        n343 = for {
          tunnel: [w694] -> w685 mode=indexing
          tunnel: w686 -> [w693] mode=indexing
          n344 = call-poly <vilib>:"Waveform to XY Pairs.vi"("waveform in"=w693) -> ("XY pairs"=w697:cluster{"x":timestamp, "y":dbl}[])  [unwired: 8 in, 2 out]
          n345 = for {
            tunnel: w697 -> [w701] mode=indexing
            tunnel: [w699] -> w695 mode=indexing
            tunnel: [w698] -> w696 mode=indexing
            n346 = Unbundle(w701) -> ("x"=w700:timestamp, "y"=w699:dbl)
            n347 = To Double Precision Float(number=w700) -> (double precision float=w698:dbl)
          }
          n348 = Bundle(w696, w695) -> (w694:cluster{dbl[], dbl[]})  [unwired: 1 in]
        }
        n349 = Format Date/Time String(time format string (%c)="%Y-%m-%d", seconds (now)=w678) -> (date/time string=w676:string)  [unwired: 1 in]
        n350 = Build Path(base path=w669, name or relative path=w676) -> (appended path=w674:path)
        n351 = Build Path(base path=w674, name or relative path=w670) -> (appended path=w673:path)
        n352 = call <userlib>:"LV to ITX XY AutoPlot.vi"("filename"=w670, "path"=w673, "Notes"="Notes", "XY Array"=w685, "wavenames (.Vx, etc)"=string[] ["ch0", "ch1", "ch2", "ch3", "ch4", "ch5", "ch6", "ch7"]) -> ()  [unwired: 10 in, 1 out]
        n353 = Build Path(base path=w674, name or relative path=w671) -> (appended path=w672:path)
        n354 = local write "Save Data"(FALSE ("SAVE DATA")) -> ()
        n355 = call <userlib>:"LV to ITX XY AutoPlot.vi"("filename"=w671, "path"=w672, "Notes"="Notes", "XY Array"=w682, "wavenames (.Vx, etc)"=string[] ["FFT0", "FFT1", "FFT2", "FFT3", "FFT4", "FFT5", "FFT6", "FFT7"], "X,Y Log"=i32[] [1, 1]) -> ()  [unwired: 9 in, 1 out]
        n356 = call <vilib>:"Add State(s) to Queue__JKI_lib_State_Machine.vi"("State(s) in (\"\")"=w692) -> ("States Out"=w691:string)  [unwired: 14 in]
      }
      frame "4461: STOP TASKS" {
        w715 = refnum<k21>[] [] ("AI task")
        n357 = Unbundle By Name(w717) -> ("AI task"=w727:refnum<k21>[], "AO task"=w731:refnum<k21>[])
        n358 = local read "DAQ Type"() -> (w724:enum16{"None", "USB 4431", "PXI 446x"})
        n359 = call-poly <userlib>:"Empty Array__ogtk.vi"("Array"=w727) -> ("Empty Array?"=w726:bool)  [unwired: 8 in]
        n360 = Equal?(x=w724, y=enum16{"None", "USB 4431", "PXI 446x"}."None" ("DAQ Type")) -> (x = y?=w723:bool)
        n361 = Or(x=w723, y=w726) -> (x .or. y?=w725:bool)
        n362 = case shown="False" w725 {
          tunnel: w731 -> [w735 _]
          tunnel: w729 -> [w734 w763]
          tunnel: [w733 w763] -> w719
          tunnel: w727 -> [w732 _]
          frame False {
            n363 = disable-structure shown="Default" {
              disable-tunnel: w735 -> [w737 _]
              disable-tunnel: w734 -> [w738 _]
              disable-tunnel: [w739 _] -> w733
              disable-tunnel: w732 -> [w736 _]
              frame condition #0 (active) {
                n364 = for {
                  tunnel: w737 -> [w762] mode=indexing
                  tunnel: [w760] -> w744 mode=indexing
                  tunnel: w738 -> [w759]
                  tunnel: [w758] -> w741
                  n365 = call <vilib>:"DAQmx Stop Task.vi"("task/channels in"=w762, "error in"=w759) -> ("task out"=w760:refnum<k21>, "error out"=w758:errorcluster)  [unwired: 12 in]
                  n366 = Wait (ms)(milliseconds to wait=u32 50) -> ()  [unwired: 1 out]
                }
                n367 = for {
                  tunnel: w736 -> [w757] mode=indexing
                  tunnel: [w755] -> w740 mode=indexing
                  tunnel: w741 -> [w754]
                  tunnel: [w753] -> w743
                  n368 = call <vilib>:"DAQmx Stop Task.vi"("task/channels in"=w757, "error in"=w754) -> ("task out"=w755:refnum<k21>, "error out"=w753:errorcluster)  [unwired: 12 in]
                  n369 = Wait (ms)(milliseconds to wait=u32 50) -> ()  [unwired: 1 out]
                }
                n370 = for {
                  tunnel: w744 -> [w752] mode=indexing
                  tunnel: w743 -> [w750]
                  tunnel: [w749] -> w742
                  n371 = call <vilib>:"DAQmx Clear Task.vi"("task in"=w752, "error in"=w750) -> ("error out"=w749:errorcluster)  [unwired: 13 in]
                  n372 = Wait (ms)(milliseconds to wait=u32 50) -> ()  [unwired: 1 out]
                }
                n373 = for {
                  tunnel: w740 -> [w748] mode=indexing
                  tunnel: w742 -> [w746]
                  tunnel: [w745] -> w739
                  n374 = call <vilib>:"DAQmx Clear Task.vi"("task in"=w748, "error in"=w746) -> ("error out"=w745:errorcluster)  [unwired: 13 in]
                  n375 = Wait (ms)(milliseconds to wait=u32 50) -> ()  [unwired: 1 out]
                }
              }
              frame condition #1 {
              }
            }
          }
          frame True {
          }
        }
        n376 = local write "RESET"(FALSE ("EXIT")) -> ()
        n377 = Bundle By Name(cluster=w717, "AI task"=w715, "AO task"=w715) -> (w716:T13)
        n378 = call <vilib>:"Add State(s) to Queue__JKI_lib_State_Machine.vi"("State(s) in (\"\")"=w730) -> ("States Out"=w714:string)  [unwired: 14 in]
        n379 = call "FGV - Trigger.vi"("error in"=w719, "Function"=enum16{"write", "read"}."write", "Trigger"=FALSE) -> ("error out"=w718:errorcluster)  [unwired: 3 in, 1 out]
      }
      frame "4461: RESET" {
        n380 = call <vilib>:"Add State(s) to Queue__JKI_lib_State_Machine.vi"("State(s) in Front (\"\")"="4461: STOP TASKS", "State(s) in (\"\")"=w768) -> ("States Out"=w764:string)  [unwired: 13 in]
      }
    }
    n381 = call "StateHistory.vi"("Current State in"=w3) -> ("Current State out"=→"Current State":string, "delimited string"=→"State History":string)  [unwired: 9 in]
  }
